vi "uA_Measurement_kit_v2_none_log.vi"() -> ()   [LabVIEW 2017]
uses:
  Range_Shunt_selector.ctl
  <vilib>/Utility/file.llb/Write Delimited Spreadsheet (string).vi
  <vilib>/Waveform/WDTFileIO.llb/ Write Waveform to File.vi
  <vilib>/Waveform/WDTFileIO.llb/Read Waveform from File.vi
  <vilib>/Utility/config.llb/Write Key (I32).vi
  <vilib>/Utility/config.llb/Write Key (Boolean).vi
  <vilib>/Utility/config.llb/Read Key (I32).vi
  <vilib>/Utility/config.llb/Read Key (Boolean).vi
  <vilib>/measure/madcrms.llb/Basic Averaged DC-RMS for 1 Chan.vi
  <resource>/objmgr/daqmx.rc
  <vilib>/Utility/config.llb/NI_LVConfig.lvlib
  <vilib>/measure/NI_MAPro.lvlib
panel:
  out "first_time":timestamp
  out "Ver":string
  out "Samples":i32=20000
  out "error out 3":errorcluster
  out "PhysicalChanName":tag
  out "DEV SN":u32 format="%.0x"
  out "mARange":dbl
  out "Boolean":bool
  out "DevSerialNum":u32
  in  "uA_bank0":dbl=1.5 format="%#_13g"
  out "Task out":refnum<k21>="Stop"
  out "Sample rate":dbl=20000.0 format="%#_13g"
  out "Clear":bool=TRUE
  out "seconds since 1Jan1904":timestamp
  in  "Tab Control":enum32{"Current Tracking", "Logging"}(tab)
  out "Total Time":i32
  in  "Sampling Rate":T1(ring)
  out "out_range":bool
  in  "Save setting":bool
  out "PW_Source":bool
  out "EX_IN_INdicator":bool
  out "Lable.Unit_VOl_MA_UA":string
  in  "Ext PW Vol Monitor":bool
  out "POWER ON_OFF":bool
  out "vbat_lb":dbl format="%#_4f"
  in  "bypass Shunt":bool
  in  "Internal PW":bool
  in  "USB":tag="Dev1"
  out "schematic":bool
  in  "Save":bool
  in  "Load":bool
  in  "Calib":bool
  in  "Power ON/OFF":bool
  in  "Profile":enum16{"SAM", "DIANA", "Hi-POWER", "Other..."}(ring)
  in  "Take Picture":bool
  in  "Orginal":bool
  in  "Clear Graph":bool
  in  "ZOOM M1M2":bool
  in  "ZOOM -":bool
  in  "ZOOM +":bool
  in  "stop":bool
  out "Vbat":dbl format="%#.3f"
  in  "Measure":bool
  in  "Range - Shunts":T2
  out "PW_Internal_Source":dbl
  out "Min":dbl
  out "Max":dbl
  out "Delta(s)":sgl
  in  "Center":bool
  out "Avg":dbl
  out "Waveform_main":waveform(sgl)(graph)
  out "Waveform_sub":waveform(dbl)(graph)
  out "Average (uA)":dbl caption="Average (mA)" format="%#_6f"
  in  "Vout  - Vbat profile":enum16{"3.8VDC", "2.9VDC", "By Pass", "4.0VDC"}(ring)=enum."2.9VDC" caption="Vout  - Vbat"
  # "Vbat"
  # "Vdut- Vbat"
  # "DUT"
  # "µPower kit for Wear OS Dev"
  # "Rs"
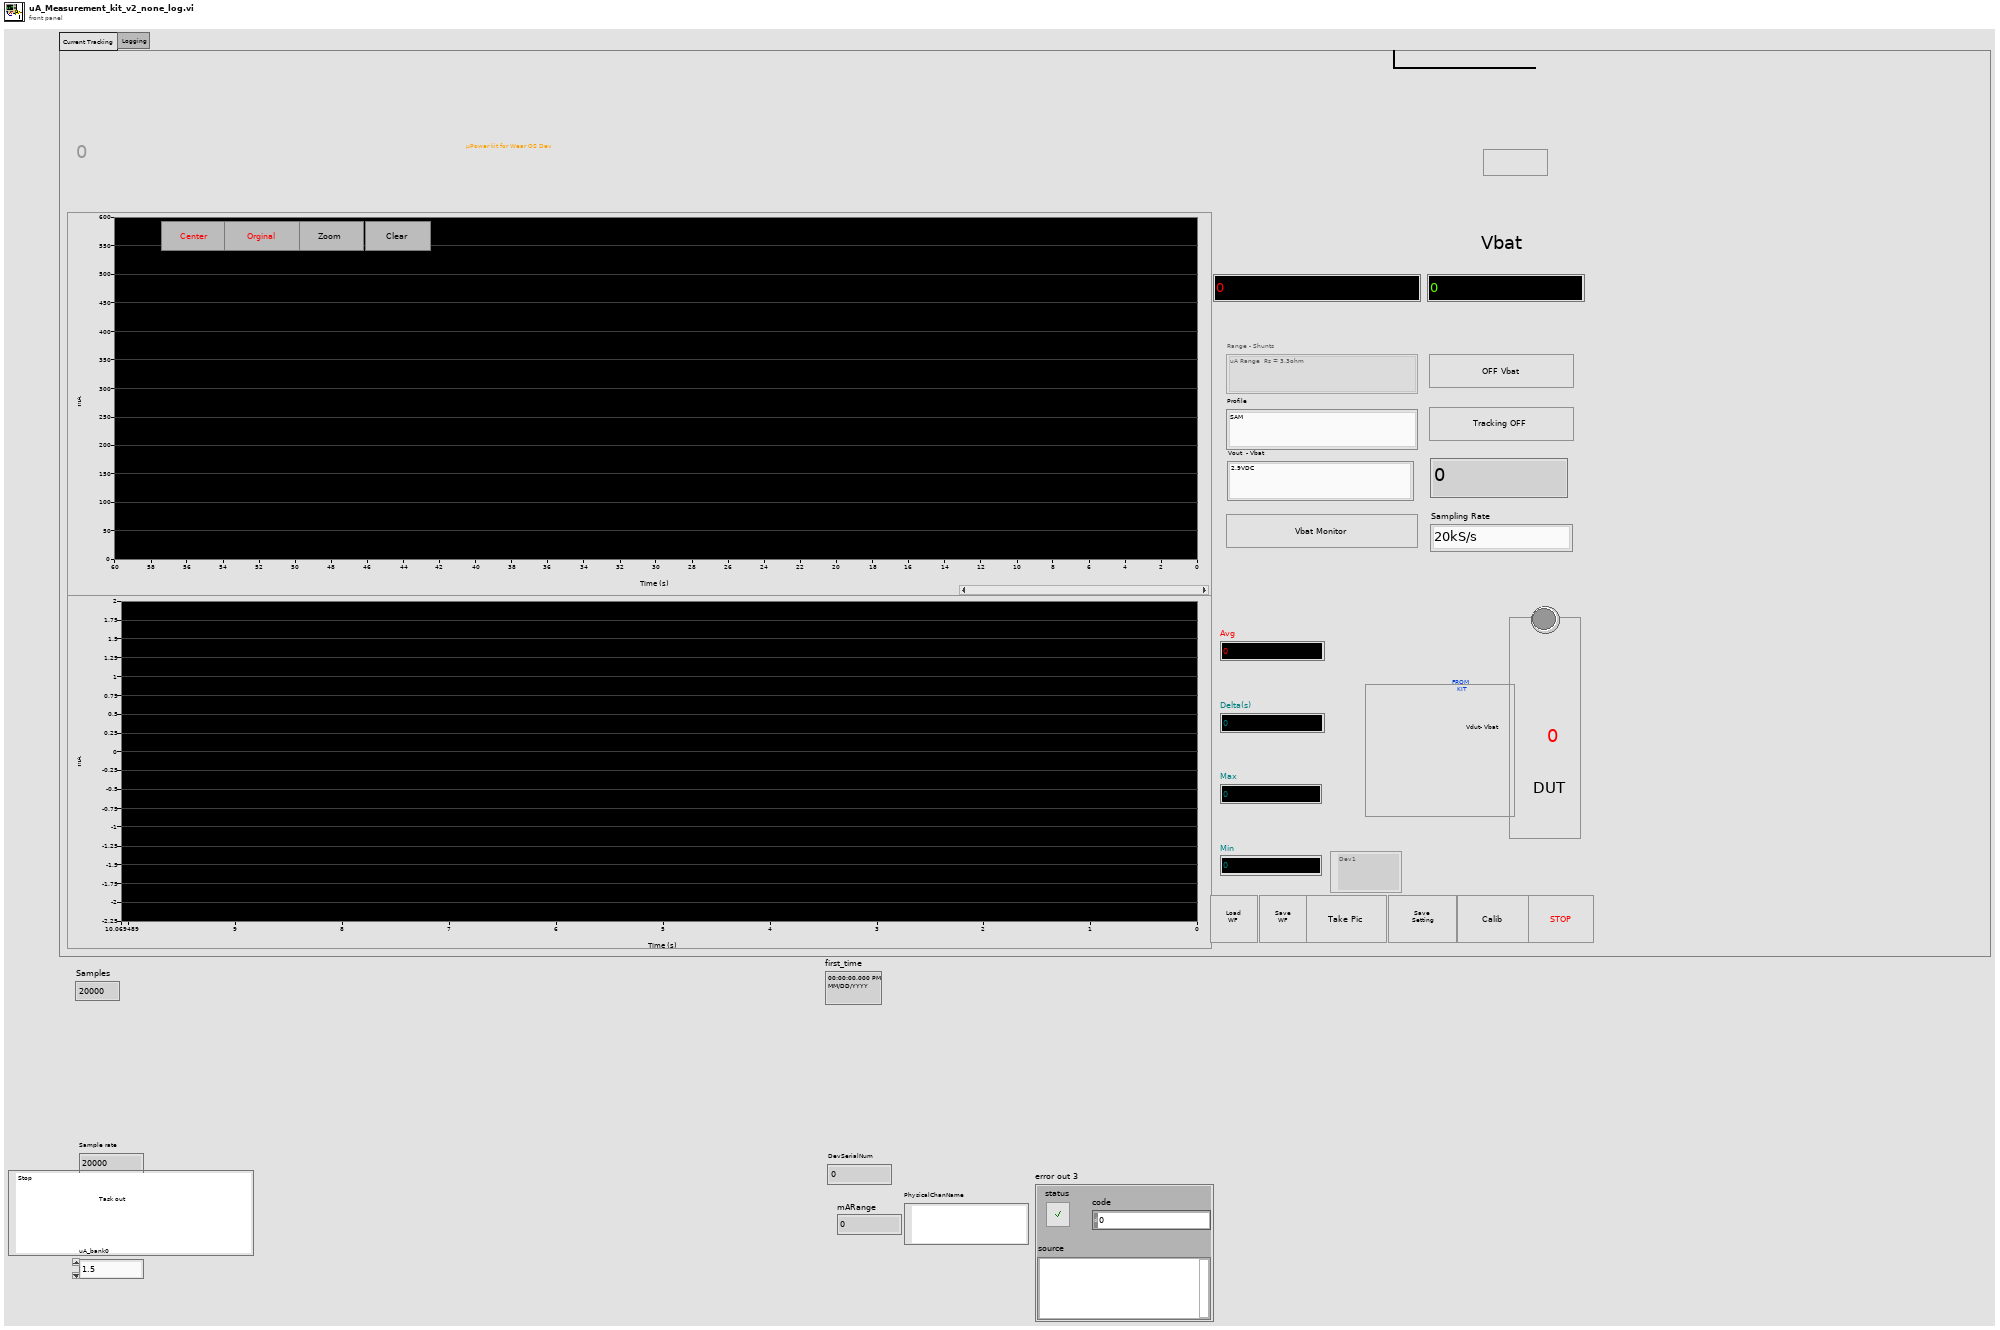
[diagram p1: front panel]
types:
  T1 = enum16{"20kS/s", "10kS/s", "5kS/s", "2kS/s", "1kS/s", "500S/s", "100S/s"}
  T2 = typedef "Range_Shunt_selector.ctl" = enum16{"uA Range  Rs = 3.3ohm", "mA Range Rs = 3.3ohm", "mA Range Rs = 1ohm", "mA Range Rs = 1ohm - X2"}
  T3 = enum8{"Enabled", "Disabled", "Disabled and Grayed Out"}
  T4 = enum16{"open", "replace", "create", "open or create", "replace or create", "replace or create with confirmation"}
  T5 = typedef "NI_LVConfig.lvlib/Config Data RefNum.ctl" = refnum<k1>
  T6 = enum16{"Internal PW Source", "External PW Source"}
  T7 = enum16{"Turn On bypass - Off Shunt", "Turn Off bypass - On Shunt"}
  T8 = typedef "LVCursorListTypeDef.ctl" = cluster{"Name":string, "Color":u32, "Style":u8, "Point Style":u8, "Name Visible":bool, "Allow Drag":bool, "Cursor Mode":u32, "Plot":i32, "Index":i32, "Position":cluster{"X":dbl, "Y":dbl}, "X Scale":u32, "Y Scale":u32, "Watch Plots":i32[], "Watch All Plots":bool, "Plot Area":i32, "Label Offset":cluster{"X":dbl, "Y":dbl}}[]
  T9 = typedef "imagedata.ctl" = cluster{"image type":i32, "image depth":i32, "image":u8[], "mask":u8[], "colors":u32[], "Rectangle":cluster{"left":i16, "top":i16, "right":i16, "bottom":i16}}
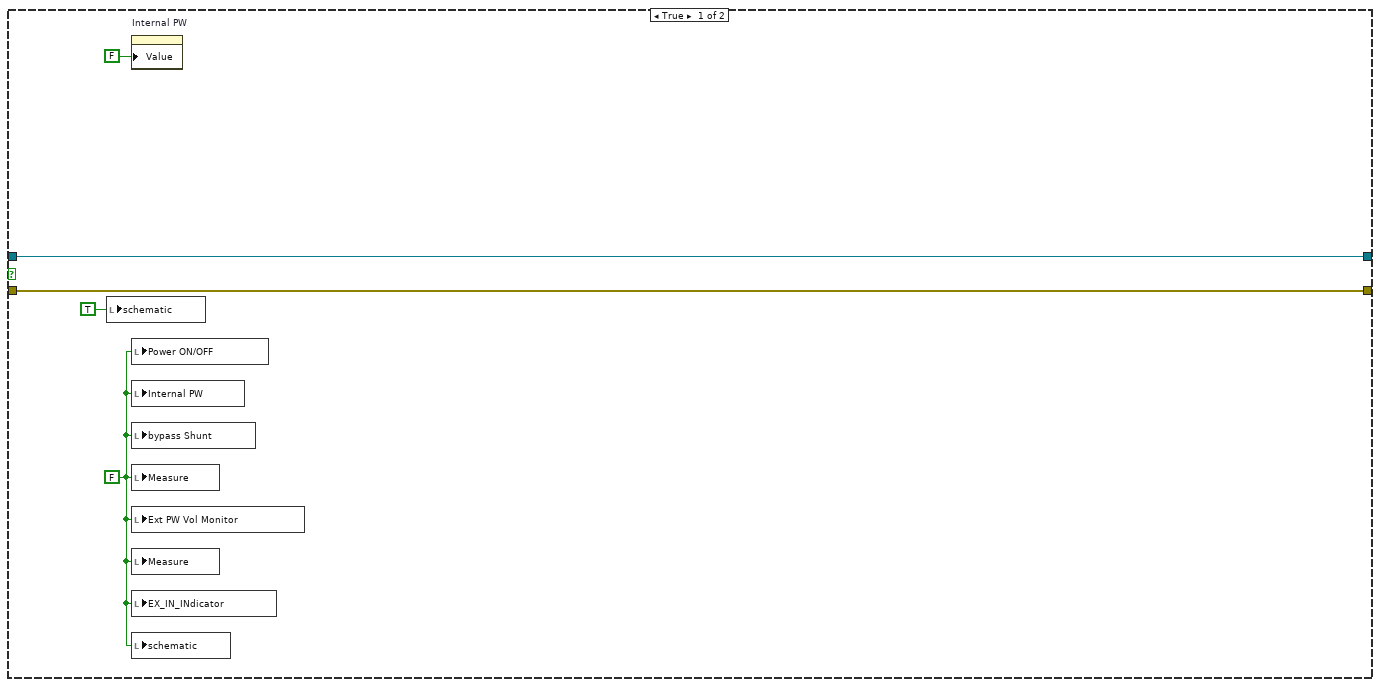
[diagram p3: hidden frame]
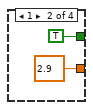
[diagram p4: hidden frame]
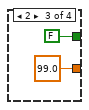
[diagram p5: hidden frame]
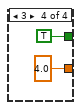
[diagram p6: hidden frame]
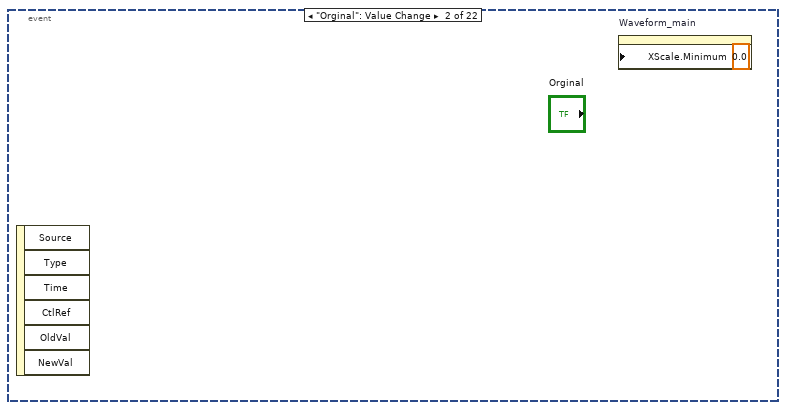
[diagram p12: hidden frame]
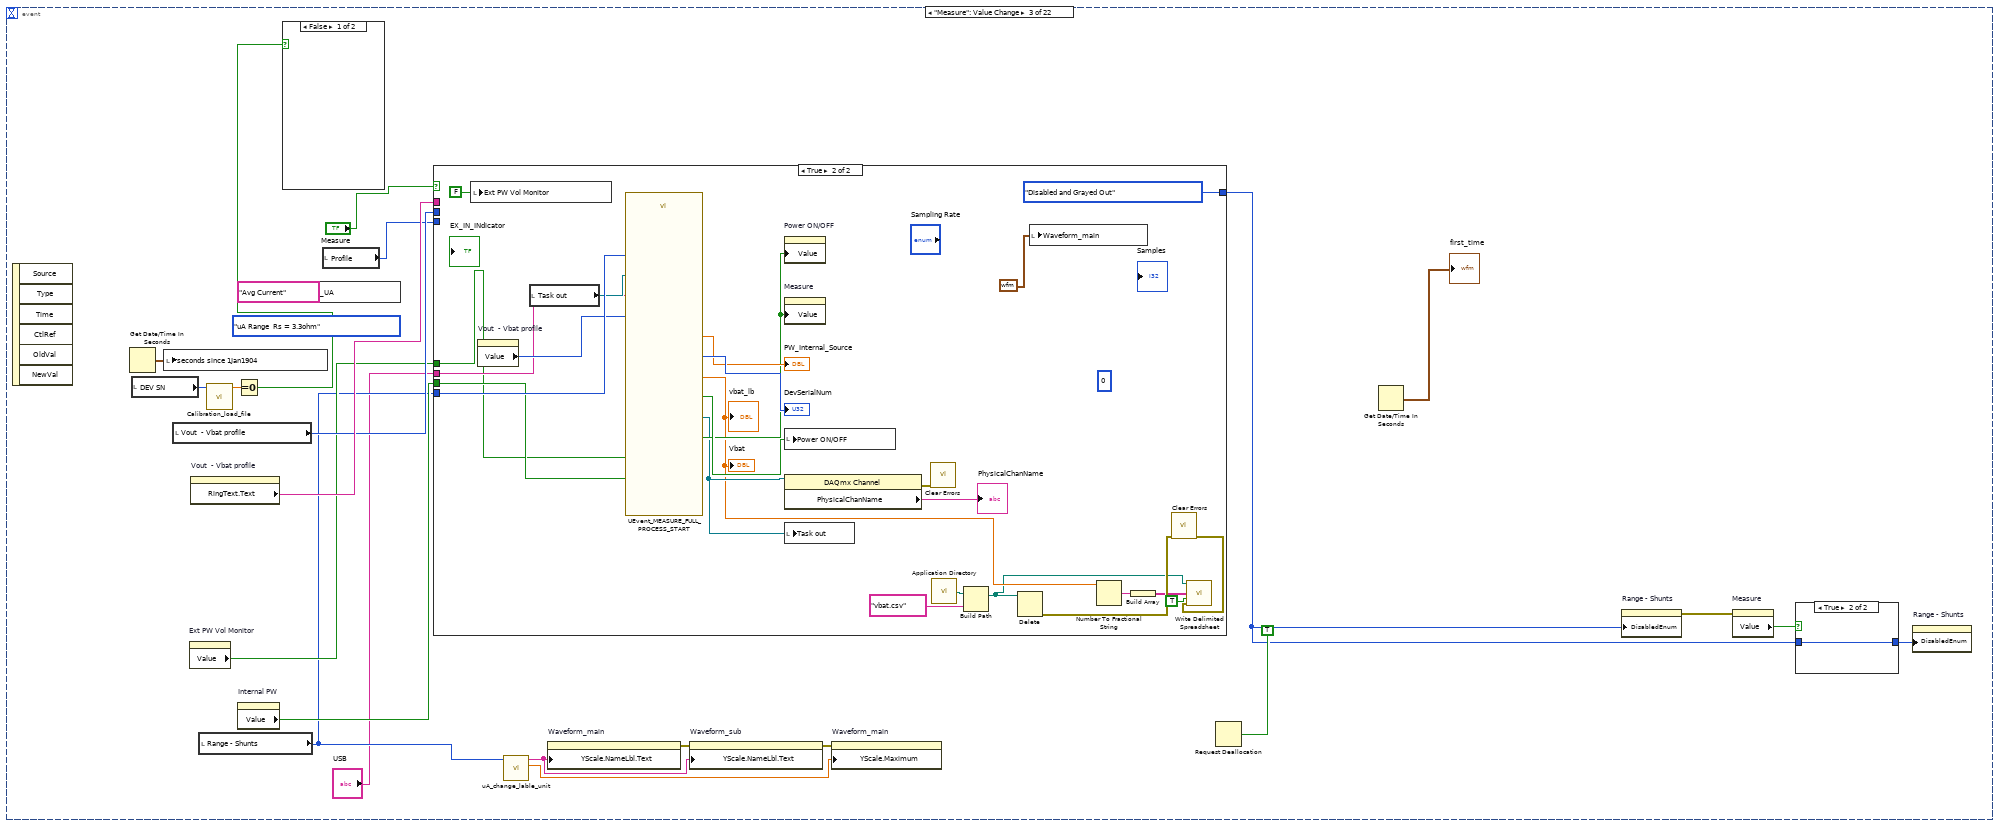
[diagram p13: hidden frame]
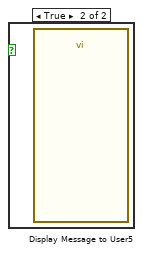
[diagram p14: hidden frame]
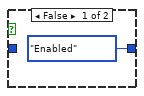
[diagram p15: hidden frame]
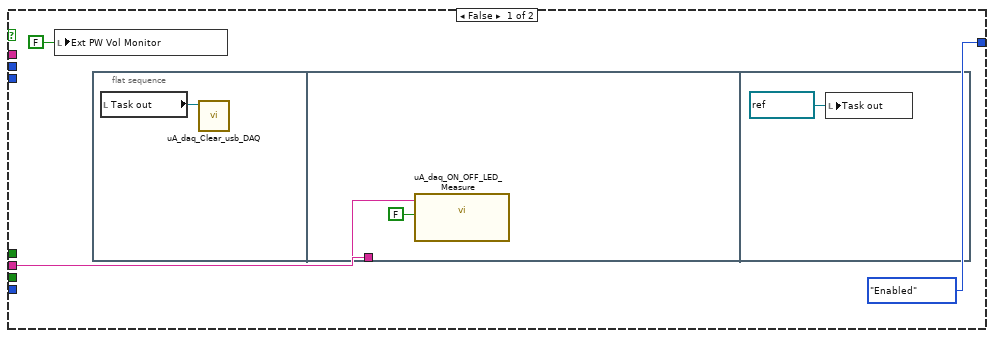
[diagram p16: hidden frame]
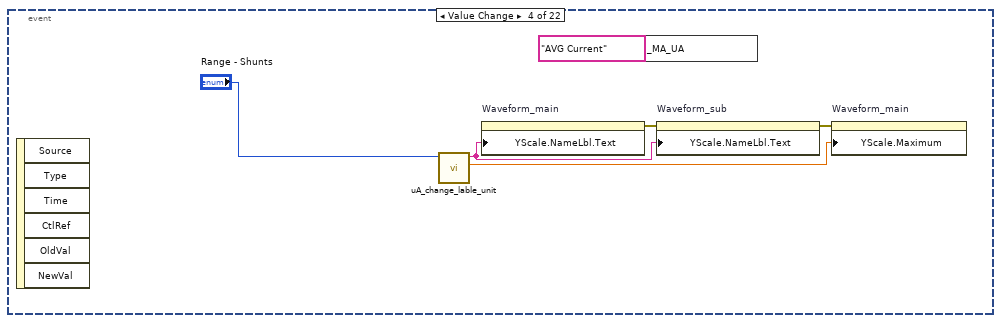
[diagram p17: hidden frame]
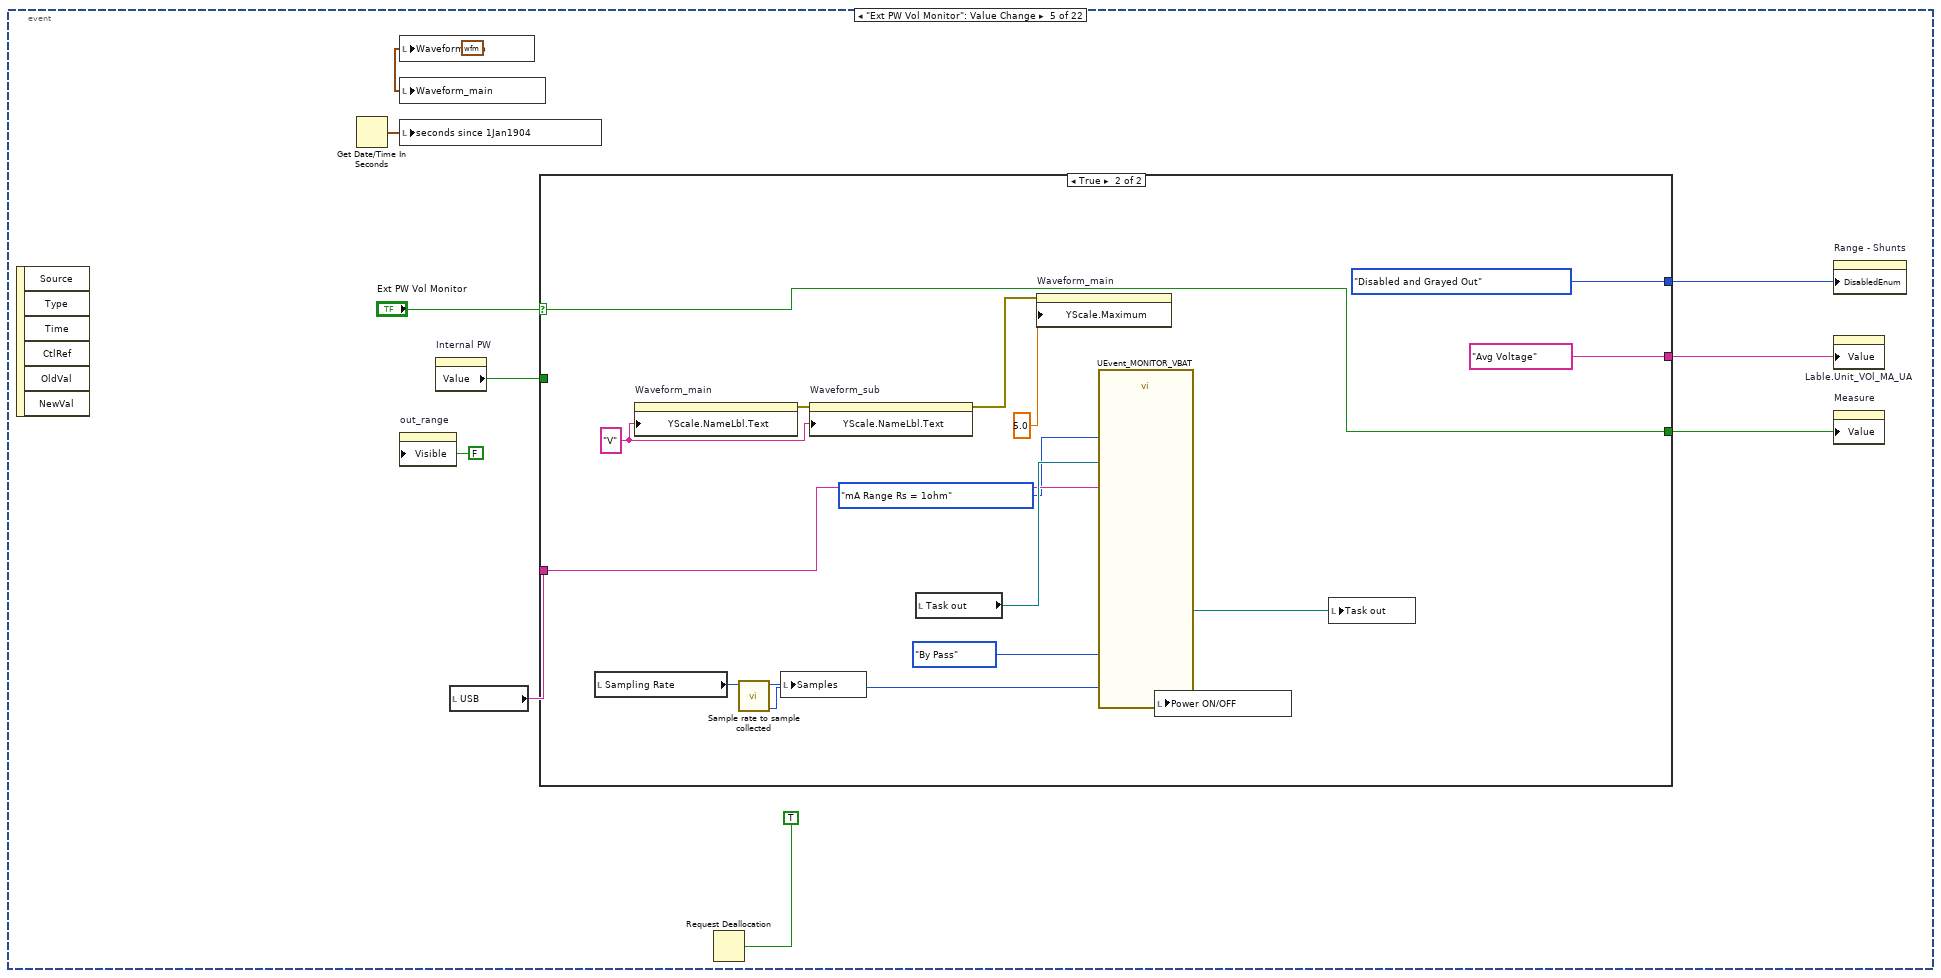
[diagram p18: hidden frame]
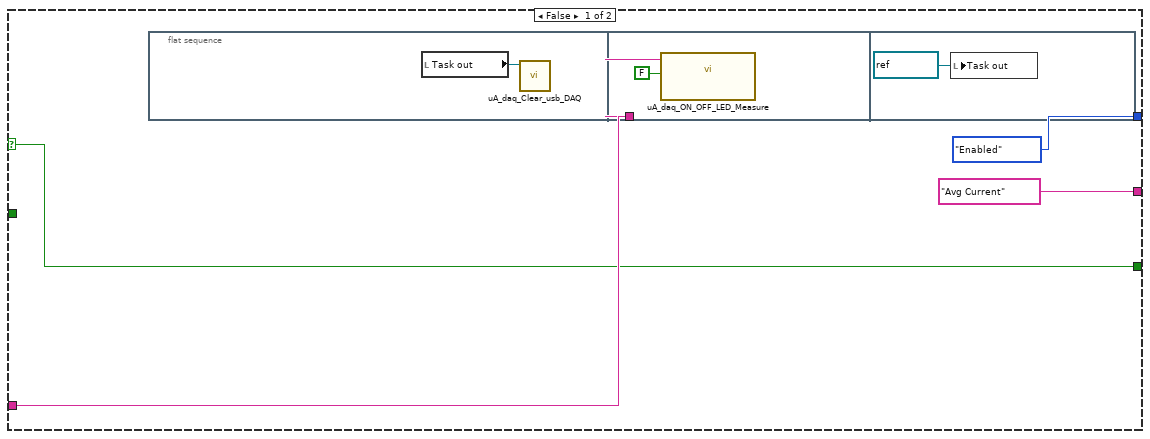
[diagram p19: hidden frame]
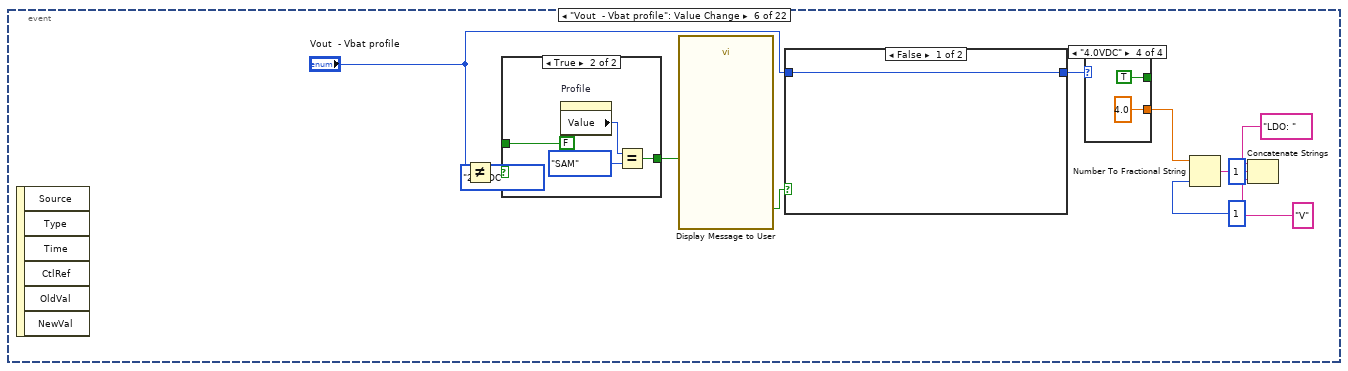
[diagram p20: hidden frame]
diagram:
  w2 = 24164516  # 1200s
  n1 = flat-sequence {
    tunnel: [w45] -> w5
    tunnel: [w48] -> w4
    frame #0 {
      w15 = TRUE ("s")
      w26 = FALSE ("Power ON/OFF")
      w45 = refnum<k21> "Stop" ("task out")
      n2 = property class="DAQmx System"() -> (error out=w39:errorcluster, "Device Names"=w40:tag[])  [unwired: 2 in, 1 out]
      n3 = property on="Range - Shunts" class="Enum (strict)"("DisabledEnum"=T3."Enabled" ("Disabled")) -> (error out=w8:errorcluster)  [unwired: 2 in, 1 out]
      n4 = local write "Vout  - Vbat profile"(enum16{"3.8VDC", "2.9VDC", "By Pass", "4.0VDC"}."By Pass" ("Vout  - Vbat profile")) -> ()
      n5 = local write "Profile"(enum16{"SAM", "DIANA", "Hi-POWER", "Other..."}."Hi-POWER" ("Profile")) -> ()
      n6 = for {
        tunnel: w40 -> [w102] mode=indexing
        shift-right: [w106] -> _
        shift-left: w39 -> [w107]
        tunnel: [w102] -> w38
        tunnel: [w101] -> w20
        stop <- w103 stop-if-true
        n7 = property class="DAQmx Device"(error in=w107, "Active Device"=w102) -> (error out=w106:errorcluster, "DevSerialNum"=w101:u32, "DevIsSimulated"=w105:bool)  [unwired: 1 in, 1 out]
        n8 = Equal?(x=w105, y=FALSE) -> (x = y?=w103:bool)
      }
      "DEV SN" <- w20
      n9 = local write "Power ON/OFF"(w26) -> ()
      n10 = local write "POWER ON_OFF"(w26) -> ()
      n11 = Select(t="Average (mA)" ("Caption.Text"), s=w15, f="Average (uA)" ("Caption.Text")) -> (s? t:f=w18:string)
      n12 = call <vilib>:"Application Directory.vi"() -> ("Application Directory"=w33:path)
      n13 = Select(t="mA" ("Caption.Text"), s=w15, f="uA" ("Caption.Text")) -> (s? t:f=w17:string)
      n14 = property on="out_range" class="Bool (strict)"(error in=w8, "Visible"=FALSE) -> (error out=w11:errorcluster)  [unwired: 1 in, 1 out]
      n15 = Build Path(base path=w33, name or relative path="Setting.cfg") -> (appended path=w31:path)
      n16 = property on="Average (uA)" class="DigNum (strict)"("Caption.Text"=w18) -> ()  [unwired: 2 in, 2 out]
      n17 = property on="Waveform_sub" class="WFGraph (strict)"("YScale.NameLbl.Text"=w17) -> ()  [unwired: 2 in, 2 out]
      n18 = property on="Waveform_main" class="WFGraph (strict)"("YScale.NameLbl.Text"=w17) -> ()  [unwired: 2 in, 2 out]
      n19 = call <vilib>:"Open Config Data.vi"("configuration file path"=w31) -> ("error out"=w27:errorcluster, "file created?"=w34:bool, "refnum"=w30:T5)  [unwired: 8 in]
      n20 = property on="Ext PW Vol Monitor" class="Bool (strict)"(error in=w11, "Value"=FALSE ("Record uA & Vbat")) -> (error out=w10:errorcluster)  [unwired: 1 in, 1 out]
      n21 = case shown="False" w34 {
        tunnel: w27 -> [w62 w92]
        tunnel: [w62 w87] -> w28
        tunnel: [w61 w86] -> w29
        tunnel: w30 -> [w61 w75]
        frame True {
          w60 = FALSE ("Measure")
          n22 = local write "schematic"(TRUE ("schematic")) -> ()
          n23 = property on="Internal PW" class="Bool (strict)"("Value"=FALSE ("Internal PW")) -> ()  [unwired: 2 in, 2 out]
          n24 = local write "Power ON/OFF"(w60) -> ()
          n25 = local write "Internal PW"(w60) -> ()
          n26 = local write "bypass Shunt"(w60) -> ()
          n27 = local write "Measure"(w60) -> ()
          n28 = local write "Ext PW Vol Monitor"(w60) -> ()
          n29 = local write "Measure"(w60) -> ()
          n30 = local write "EX_IN_INdicator"(w60) -> ()
          n31 = local write "schematic"(w60) -> ()
        }
        frame False {
          (unwired) FALSE ("Visible")
          w63 = TRUE
          w76 = "SETTING" ("section")
          n32 = Not(x=w63) -> ()  [unwired: 1 out]
          n33 = local write "Internal PW"(w63) -> ()
          n34 = local write "EX_IN_INdicator"(w63) -> ()
          n35 = local write "Vout  - Vbat profile"(enum16{"3.8VDC", "2.9VDC", "By Pass", "4.0VDC"}."By Pass" ("Vout  - Vbat profile")) -> ()
          n36 = local write "Profile"(enum16{"SAM", "DIANA", "Hi-POWER", "Other..."}."Hi-POWER" ("Profile")) -> ()
          n37 = call-poly <vilib>:"Read Key.vi"("section"=w76, "error in (no error)"=w92, "key"="Range - Shunts", "refnum"=w75) -> ("error out"=w91:errorcluster, "refnum out"=w78:T5)  [unwired: 4 in, 2 out]
          n38 = local write "Range - Shunts"(Range_Shunt_selector."mA Range Rs = 1ohm" ("Range - Shunts")) -> ()
          n39 = call-poly <vilib>:"Read Key.vi"("section"=w76, "error in (no error)"=w91, "key"="Profile", "refnum"=w78) -> ("error out"=w90:errorcluster, "refnum out"=w77:T5)  [unwired: 4 in, 2 out]
          n40 = call-poly <vilib>:"Read Key.vi"("section"=w76, "error in (no error)"=w90, "key"="Vout  - Vbat profile", "refnum"=w77) -> ("error out"=w89:errorcluster, "value"=w67:i32, "refnum out"=w79:T5)  [unwired: 4 in, 1 out]
          n41 = case shown="0, Default" w67 {
            tunnel: [3.8 2.9 99.0 4.0] -> w71
            tunnel: [TRUE ("Visible") TRUE ("Visible") FALSE ("Visible") TRUE ("Visible")] -> _
            frame 0, Default {
            }
            frame 1 {
            }
            frame 2 {
            }
            frame 3 {
            }
          }
          n42 = call-poly <vilib>:"Read Key.vi"("section"=w76, "error in (no error)"=w89, "key"="Internal PW", "refnum"=w79) -> ("error out"=w88:errorcluster, "refnum out"=w80:T5)  [unwired: 4 in, 2 out]
          n43 = call-poly <vilib>:"Read Key.vi"("section"=w76, "error in (no error)"=w88, "key"="bypass Shunt", "refnum"=w80) -> ("error out"=w87:errorcluster, "value"=w74:bool, "refnum out"=w86:T5)  [unwired: 4 in, 1 out]
          n44 = local write "bypass Shunt"(w74) -> ()
          n45 = Number To Fractional String(number=w71, width (-)=i16 1, precision (6)=i16 1) -> (F-format string=w68:string)  [unwired: 1 in]
          n46 = Concatenate Strings("LDO: " ("string"), w68, "V" ("string")) -> ()  [unwired: 1 out]
        }
      }
      n47 = local write "USB"(w38) -> ()
      n48 = property on="out_range" class="Bool (strict)"(error in=w10, "Visible"=FALSE) -> (error out=w9:errorcluster)  [unwired: 1 in, 1 out]
      n49 = call "Calibration_load_file.vi"("DEV SN"=w20) -> ("Calib value-mA"=→"mARange":dbl, "Calib value-uA"=w21:dbl)  [unwired: 8 in]
      n50 = local write "uA_bank0"(w21) -> ()
      n51 = call <vilib>:"Application Directory.vi"() -> ("Application Directory"=w47:path)
      n52 = call "uA_build_version.vi"("error in (no error)"=w9, "name or relative path"="uPower_kit_wear_os.exe", "path"=w47) -> ("error out"=w44:errorcluster, "FileVersion"=w43:string)  [unwired: 6 in, 1 out]
      n53 = case shown="Error" w44 {
        selector: w44 -> [_ w110]
        tunnel: w43 -> [w108 _]
        tunnel: [w108 "" ("FileVersion")] -> w42
        frame No Error {
        }
        frame Error {
          n54 = call <vilib>:"Clear Errors.vi"("error in (no error)"=w110) -> ()  [unwired: 5 in, 2 out]
        }
      }
      "Ver" <- w42
      n55 = local write "Measure"(FALSE ("Measure")) -> ()
      n56 = local write "schematic"(TRUE ("schematic")) -> ()
      n57 = disable-structure shown="Disabled" {
        frame Disabled {
          n58 = call <vilib>:"Application Directory.vi"() -> ("Application Directory"=w57:path)
          n59 = Build Path(base path=w57, name or relative path="datalog.dlog" ("pattern label")) -> (appended path=w55:path)
          n60 = Open/Create/Replace File(file path (use dialog)=w55, operation (0:open)=T4."replace or create", access (0:read/write)=enum16{"read/write", "read-only", "write-only"}."write-only") -> ()  [unwired: 3 in, 3 out]
        }
        frame Enabled {
        }
      }
      n61 = call <vilib>:"Close Config Data.vi"("error in (no error)"=w28, "refnum"=w29) -> ()  [unwired: 8 in, 2 out]
      n62 = Obtain Queue(name (unnamed)="Data", element data type=waveform(sgl) {"t0"=timestamp(0 s since 1904-01-01), "dt"=1.0, "Y"=[]} ("Waveform Chart 2")) -> (queue out=w48:refnum<queue>)  [unwired: 3 in, 2 out]
      "Clear" <- FALSE ("Clear")
      "Sample rate" <- 20000.0 ("Sample rate")
      "Task out" <- w45
    }
  }
  n63 = Multiply(x=w2, y=4) -> (x*y=w1:i32)
  n64 = while {
    stop <- FALSE stop-if-true
    n65 = event shown="[0] Timeout" {
      selector: _ -> [_ _ _ _ _ _ _ _ _ _ _ _ _ _ _ _ _ _ _ _ _ _]
      dyn-events: _ -> [_ _ _ _ _ _ _ _ _ _ _ _ _ _ _ _ _ _ _ _ _ _]
      timeout: 400 -> [_ _ _ _ _ _ _ _ _ _ _ _ _ _ _ _ _ _ _ _ _ _]
      event Timeout {
        n66 = event-data() -> ()  [unwired: 1 in, 3 out]
        n67 = disable-structure shown="Disabled" {
          frame Disabled {
            n68 = local read "Task out"() -> (w114:refnum<k21>)
            n69 = Equal?(x=w114, y=refnum<k21> "Stop") -> (x = y?=w115:bool)
            n70 = case shown="False" w115 {
              frame True {
              }
              frame False {
                n71 = local read "seconds since 1Jan1904"() -> (w120:timestamp)
                n72 = local read "first_time"() -> (w118:timestamp)
                n73 = Get Date/Time In Seconds() -> (seconds since 1Jan1904=w119:timestamp)
                n74 = Subtract(x=w119, y=w118) -> (x-y=→"Total Time":dbl)
                n75 = Subtract(x=w119, y=w120) -> (x-y=w123:dbl)
                n76 = Greater Or Equal?(x=w123, y=60.0) -> (x >= y?=w121:bool)
                n77 = case shown="True" w121 {
                  tunnel: w119 -> [_ _]
                  frame False {
                  }
                  frame True {
                    w140 = 5 items=["verify"=2, "reserve"=4, "commit"=3, "unreserve"=5, "abort"=6] ("action")
                    n78 = Get Date/Time In Seconds() -> (seconds since 1Jan1904=→"seconds since 1Jan1904":timestamp)
                    n79 = local read "Task out"() -> (w154:refnum<k21>)
                    n80 = call <vilib>:"DAQmx Stop Task.vi"("task/channels in"=w154) -> ("task out"=w144:refnum<k21>, "error out"=w142:errorcluster)  [unwired: 13 in]
                    n81 = call <vilib>:"DAQmx Control Task.vi"("task/channels in"=w144, "action"=w140, "error in"=w142) -> ("task out"=w143:refnum<k21>, "error out"=w141:errorcluster)  [unwired: 11 in]
                    n82 = call <vilib>:"DAQmx Clear Task.vi"("task in"=w143, "error in"=w141) -> ("error out"=w136:errorcluster)  [unwired: 13 in]
                    n83 = case shown="No Error" w136 {
                      selector: w136 -> [w157 w159]
                      tunnel: [w157 w159] -> w135
                      frame No Error {
                        n84 = Wait (ms)(milliseconds to wait=u32 100) -> ()  [unwired: 1 out]
                        n85 = local write "Task out"(refnum<k21> "Stop" ("Task out")) -> ()
                      }
                      frame Error {
                      }
                    }
                    n86 = local read "USB"() -> (w146:tag)
                    n87 = call <vilib>:"Clear Errors.vi"("error in (no error)"=w135) -> ("error out"=w153:errorcluster)  [unwired: 5 in, 1 out]
                    n88 = property on="Range - Shunts" class="Enum (strict)"() -> ("Value"=w150:T2)  [unwired: 2 in, 2 out]
                    n89 = call "uA_daq_Read_Battery_Voltage.vi"("error in"=w153, "USB DAQ"=w146) -> ("error out"=w151:errorcluster, "Battery_Voltage"=w152:dbl)  [unwired: 8 in]
                    n90 = local write "PW_Internal_Source"(w152) -> ()
                    n91 = call "uA_daq_Read_DUT_Voltage.vi"("error in"=w151, "USB DAQ"=w146) -> ("error out"=w139:errorcluster, "DUT_Voltage"=w124:dbl)  [unwired: 8 in]
                    n92 = local write "Vbat"(w124) -> ()
                    n93 = call <vilib>:"Application Directory.vi"() -> ("Application Directory"=w129:path)
                    n94 = Number To Fractional String(number=w124) -> (F-format string=w126:string)  [unwired: 3 in]
                    n95 = Build Path(base path=w129, name or relative path="vbat.csv" ("pattern label")) -> (appended path=w128:path)
                    n96 = Build Array(w126) -> (w125:string[])
                    n97 = local read "Sampling Rate"() -> (w132:T1)
                    n98 = property on="Ext PW Vol Monitor" class="Bool (strict)"() -> ("Value"=w147:bool)  [unwired: 2 in, 2 out]
                    n99 = call-poly <vilib>:"Write Delimited Spreadsheet.vi"("file path (dialog if empty)"=w128, "1D data"=w125, "append to file? (new file:F)"=TRUE) -> ()  [unwired: 11 in, 2 out]
                    n100 = call "Sample rate to sample collected.vi"("Sampling Rate _menu"=w132) -> ("Sample_rate"=w131:u32, "Sample"=w133:i32)  [unwired: 9 in]
                    n101 = for {
                      N: 3 -> [_]
                      tunnel: w150 -> [w167]
                      tunnel: [w166] -> w149
                      tunnel: w146 -> [w165]
                      tunnel: enum16{"Streaming", "Read All", "Stop"}."Streaming" ("Acquire Mode") -> [w163]
                      tunnel: w139 -> [w164]
                      tunnel: [w162] -> w145
                      tunnel: w131 -> [w160]
                      stop <- w161 continue-if-true
                      n102 = call "uA_daq_Re_Init_daq_follow_input.vi"("rate"=w160, "error in (no error)"=w164, "Acquire Mode"=w163, "USB"=w165, "Range_shunt"=w167) -> ("error out"=w162:errorcluster, "Refnum out"=w166:refnum<k21>)  [unwired: 5 in]
                      n103 = Unbundle By Name(w162) -> ("status"=w161:bool)
                    }
                    n104 = local write "Samples"(w133) -> ()
                    n105 = call "uA_DAQ_Init_Monitor_Stream_vbat_selector.vi"("Sample rate"=w131, "error in (no error)"=w145, "USB"=w146, "Ext PW Vol Monitor"=w147, "Refnum in"=w149) -> ("error out"=w134:errorcluster, "Refnum out"=w148:refnum<k21>)  [unwired: 5 in]
                    n106 = call <vilib>:"Clear Errors.vi"("error in (no error)"=w134) -> ()  [unwired: 5 in, 2 out]
                    n107 = local write "Task out"(w148) -> ()
                  }
                }
              }
            }
          }
          frame Enabled {
          }
        }
        n108 = local read "Vbat"() -> (w113:dbl)
        n109 = local write "vbat_lb"(w113) -> ()
      }
      event "Orginal": Value Change {
        n110 = event-data() -> ()  [unwired: 1 in, 6 out]
        n111 = property on="Waveform_main" class="WFGraph (strict)"("XScale.Minimum"=0.0 ("X Scale.Range:Minimum")) -> ()  [unwired: 2 in, 2 out]
      }
      event "Measure": Value Change {
        (unwired) Range_Shunt_selector."uA Range  Rs = 3.3ohm" ("Range - Shunts")
        n112 = event-data() -> ()  [unwired: 1 in, 6 out]
        n113 = Get Date/Time In Seconds() -> (seconds since 1Jan1904=w190:timestamp)
        n114 = local read "DEV SN"() -> (w172:u32)
        n115 = local write "seconds since 1Jan1904"(w190) -> ()
        n116 = local read "Vout  - Vbat profile"() -> (w187:enum16{"3.8VDC", "2.9VDC", "By Pass", "4.0VDC"})
        n117 = property on="Ext PW Vol Monitor" class="Bool (strict)"() -> ("Value"=w180:bool)  [unwired: 2 in, 2 out]
        n118 = property on="Vout  - Vbat profile" class="Enum (strict)"() -> ("RingText.Text"=w188:string)  [unwired: 2 in, 2 out]
        n119 = local read "Range - Shunts"() -> (w178:T2)
        n120 = call "Calibration_load_file.vi"("DEV SN"=w172) -> ("Calib value-uA"=w171:dbl)  [unwired: 8 in, 1 out]
        n121 = Equal To 0?(x=w171) -> (x = 0?=w170:bool)
        n122 = property on="Internal PW" class="Bool (strict)"() -> ("Value"=w181:bool)  [unwired: 2 in, 2 out]
        n123 = local write "Lable.Unit_VOl_MA_UA"("Avg Current" ("Lable.Unit_VOl_MA_UA")) -> ()
        n124 = case shown="False" w170 {
          frame False {
          }
          frame True {
            n125 = call "Display Message to User5"() -> ()  [unwired: 10 in, 2 out]
          }
        }
        n126 = local read "Profile"() -> (w186:enum16{"SAM", "DIANA", "Hi-POWER", "Other..."})
        n127 = case shown="True" "Measure" {
          tunnel: w188 -> [_ _]
          tunnel: w187 -> [_ _]
          tunnel: w186 -> [_ _]
          tunnel: w178 -> [_ w222]
          tunnel: w181 -> [_ w219]
          tunnel: "USB" -> [w195 w217]
          tunnel: w180 -> [_ w214]
          tunnel: [T3."Enabled" ("Disabled") T3."Disabled and Grayed Out" ("Disabled")] -> w174
          frame False {
            n128 = local write "Ext PW Vol Monitor"(FALSE ("Ext PW Vol Monitor")) -> ()
            n129 = flat-sequence {
              tunnel: w195 -> [w199]
              frame #0 {
                n130 = local read "Task out"() -> (w197:refnum<k21>)
                n131 = call "uA_daq_Clear_usb_DAQ.vi"("Refnum in"=w197) -> ()  [unwired: 11 in]
              }
              frame #1 {
                n132 = call "uA_daq_ON_OFF_LED_Measure.vi"("LED_meas"=FALSE ("Boolean"), "USB"=w199) -> ()  [unwired: 9 in, 1 out]
              }
              frame #2 {
                n133 = local write "Task out"(refnum<k21> "Stop" ("Refnum out")) -> ()
              }
            }
          }
          frame True {
            (unwired) u16 0 ("File_Record")
            n134 = local write "Ext PW Vol Monitor"(FALSE ("Ext PW Vol Monitor")) -> ()
            n135 = property on="Vout  - Vbat profile" class="Enum (strict)"() -> ("Value"=w220:enum16{"3.8VDC", "2.9VDC", "By Pass", "4.0VDC"})  [unwired: 2 in, 2 out]
            n136 = local read "Task out"() -> (w221:refnum<k21>)
            n137 = call "UEvent_MEASURE_FULL_PROCESS_START.vi"("Refnum in"=w221, "Range - Shunts"=w222, "Ext PW Vol Monitor"=w214, "USB"=w217, "Internal/external Power"=w219, "Vout  - Vbat profile"=w220) -> ("DevSerialNum"=→"DevSerialNum":u32, "Power ON/OFF"=w224:bool, "Refnum out"=w216:refnum<k21>, "Battery_Voltage"=→"PW_Internal_Source":dbl, "DUT_Voltage"=w203:dbl, "Measure indicator"=w218:bool)  [unwired: 3 in, 1 out]
            "Vbat" <- w203
            "vbat_lb" <- w203
            n138 = property on="Power ON/OFF" class="Bool (strict)"("Value"=w218) -> ()  [unwired: 2 in, 2 out]
            n139 = property on="Measure" class="Bool (strict)"("Value"=w218) -> ()  [unwired: 2 in, 2 out]
            n140 = local write "Power ON/OFF"(w224) -> ()
            n141 = property class="DAQmx Channel"(reference=w216) -> (error out=w213:errorcluster, "PhysicalChanName"=→"PhysicalChanName":tag)  [unwired: 1 in, 1 out]
            n142 = local write "Task out"(w216) -> ()
            n143 = call <vilib>:"Clear Errors.vi"("error in (no error)"=w213) -> ()  [unwired: 5 in, 2 out]
            n144 = call <vilib>:"Application Directory.vi"() -> ("Application Directory"=w209:path)
            n145 = Build Path(base path=w209, name or relative path="vbat.csv" ("pattern label")) -> (appended path=w202:path)
            n146 = Delete(path (use dialog)=w202) -> (error out=w210:errorcluster)  [unwired: 4 in, 2 out]
            n147 = local write "Waveform_main"(waveform(dbl) {"t0"=timestamp(0 s since 1904-01-01), "dt"=1.0, "Y"=[]} ("Waveform")) -> ()
            n148 = Number To Fractional String(number=w203) -> (F-format string=w206:string)  [unwired: 3 in]
            n149 = Build Array(w206) -> (w205:string[])
            n150 = call <vilib>:"Clear Errors.vi"("error in (no error)"=w210) -> ("error out"=w201:errorcluster)  [unwired: 5 in, 1 out]
            n151 = call-poly <vilib>:"Write Delimited Spreadsheet.vi"("file path (dialog if empty)"=w202, "1D data"=w205, "append to file? (new file:F)"=TRUE, "error in (no error)"=w201) -> ()  [unwired: 10 in, 2 out]
          }
        }
        n152 = call "uA_change_lable_unit.vi"("Range - Shunts"=w178) -> ("Y_scale"=w183:dbl, "unit"=w182:string)  [unwired: 8 in, 1 out]
        n153 = property on="Waveform_main" class="WFGraph (strict)"("YScale.NameLbl.Text"=w182) -> (error out=w185:errorcluster)  [unwired: 2 in, 1 out]
        n154 = property on="Waveform_sub" class="WFGraph (strict)"(error in=w185, "YScale.NameLbl.Text"=w182) -> (error out=w184:errorcluster)  [unwired: 1 in, 1 out]
        n155 = property on="Waveform_main" class="WFGraph (strict)"(error in=w184, "YScale.Maximum"=w183) -> ()  [unwired: 1 in, 2 out]
        n156 = Request Deallocation(TRUE ("flag")) -> ()
        n157 = Get Date/Time In Seconds() -> (seconds since 1Jan1904=→"first_time":timestamp)
        n158 = property on="Range - Shunts" class="Enum (strict)"("DisabledEnum"=w174) -> (error out=w177:errorcluster)  [unwired: 2 in, 1 out]
        n159 = property on="Measure" class="Bool (strict)"(error in=w177) -> ("Value"=w176:bool)  [unwired: 1 in, 2 out]
        n160 = case shown="True" w176 {
          tunnel: [T3."Enabled" ("Disabled") w193] -> w175
          tunnel: w174 -> [_ w193]
          frame False {
          }
          frame True {
          }
        }
        n161 = property on="Range - Shunts" class="Enum (strict)"("DisabledEnum"=w175) -> ()  [unwired: 2 in, 2 out]
      }
      event Value Change {
        n162 = event-data() -> ()  [unwired: 1 in, 6 out]
        n163 = call "uA_change_lable_unit.vi"("Range - Shunts"="Range - Shunts") -> ("Y_scale"=w229:dbl, "unit"=w228:string)  [unwired: 8 in, 1 out]
        n164 = property on="Waveform_main" class="WFGraph (strict)"("YScale.NameLbl.Text"=w228) -> (error out=w231:errorcluster)  [unwired: 2 in, 1 out]
        n165 = local write "Lable.Unit_VOl_MA_UA"("AVG Current" ("Lable.Unit_VOl_MA_UA")) -> ()
        n166 = property on="Waveform_sub" class="WFGraph (strict)"(error in=w231, "YScale.NameLbl.Text"=w228) -> (error out=w230:errorcluster)  [unwired: 1 in, 1 out]
        n167 = property on="Waveform_main" class="WFGraph (strict)"(error in=w230, "YScale.Maximum"=w229) -> ()  [unwired: 1 in, 2 out]
      }
      event "Ext PW Vol Monitor": Value Change {
        w234 = waveform(sgl) {"t0"=timestamp(0 s since 1904-01-01), "dt"=1.0, "Y"=[]} ("Waveform_main")
        n168 = event-data() -> ()  [unwired: 1 in, 6 out]
        n169 = Get Date/Time In Seconds() -> (seconds since 1Jan1904=w240:timestamp)
        n170 = local write "Waveform_sub"(w234) -> ()
        n171 = local write "Waveform_main"(w234) -> ()
        n172 = local write "seconds since 1Jan1904"(w240) -> ()
        n173 = property on="out_range" class="Bool (strict)"("Visible"=FALSE) -> ()  [unwired: 2 in, 2 out]
        n174 = property on="Internal PW" class="Bool (strict)"() -> ("Value"=w239:bool)  [unwired: 2 in, 2 out]
        n175 = local read "USB"() -> (w237:tag)
        n176 = case shown="True" "Ext PW Vol Monitor" {
          selector: "Ext PW Vol Monitor" -> [w244 w262]
          tunnel: w239 -> [_ _]
          tunnel: w237 -> [w245 w263]
          tunnel: [w244 w262] -> w236
          tunnel: ["Avg Current" ("Lable.Unit_VOl_MA_UA") "Avg Voltage" ("Lable.Unit_VOl_MA_UA")] -> w235
          tunnel: [T3."Enabled" ("Disabled") T3."Disabled and Grayed Out" ("Disabled")] -> w233
          frame False {
            n177 = flat-sequence {
              tunnel: w245 -> [w248]
              frame #0 {
                n178 = local read "Task out"() -> (w246:refnum<k21>)
                n179 = call "uA_daq_Clear_usb_DAQ.vi"("Refnum in"=w246) -> ()  [unwired: 11 in]
              }
              frame #1 {
                n180 = call "uA_daq_ON_OFF_LED_Measure.vi"("LED_meas"=FALSE ("Boolean"), "USB"=w248) -> ()  [unwired: 9 in, 1 out]
              }
              frame #2 {
                n181 = local write "Task out"(refnum<k21> "Stop" ("Refnum out")) -> ()
              }
            }
          }
          frame True {
            w261 = "V" ("Y Scale.Name Label.Text")
            n182 = local read "Sampling Rate"() -> (w253:T1)
            n183 = property on="Waveform_main" class="WFGraph (strict)"("YScale.NameLbl.Text"=w261) -> (error out=w258:errorcluster)  [unwired: 2 in, 1 out]
            n184 = call "Sample rate to sample collected.vi"("Sampling Rate _menu"=w253) -> ("Sample_rate"=w252:u32, "Sample"=w254:i32)  [unwired: 9 in]
            n185 = local write "Samples"(w254) -> ()
            n186 = property on="Waveform_sub" class="WFGraph (strict)"(error in=w258, "YScale.NameLbl.Text"=w261) -> (error out=w259:errorcluster)  [unwired: 1 in, 1 out]
            n187 = local read "Task out"() -> (w264:refnum<k21>)
            n188 = property on="Waveform_main" class="WFGraph (strict)"(error in=w259, "YScale.Maximum"=5.0 ("Y Scale.Range:Maximum")) -> ()  [unwired: 1 in, 2 out]
            n189 = call "UEvent_MONITOR_VBAT.vi"("Vout  - Vbat profile"=enum16{"3.8VDC", "2.9VDC", "By Pass", "4.0VDC"}."By Pass", "Sample rate"=w252, "USB"=w263, "Range - Shunts"=Range_Shunt_selector."mA Range Rs = 1ohm", "Refnum in"=w264) -> ("Refnum out"=w256:refnum<k21>, "Power ON/OFF"=w265:bool)  [unwired: 1 in, 4 out]
            n190 = local write "Power ON/OFF"(w265) -> ()
            n191 = local write "Task out"(w256) -> ()
          }
        }
        n192 = Request Deallocation(TRUE ("flag")) -> ()
        n193 = property on="Range - Shunts" class="Enum (strict)"("DisabledEnum"=w233) -> ()  [unwired: 2 in, 2 out]
        n194 = property on="Lable.Unit_VOl_MA_UA" class="Str"("Value"=w235) -> ()  [unwired: 2 in, 2 out]
        n195 = property on="Measure" class="Bool (strict)"("Value"=w236) -> ()  [unwired: 2 in, 2 out]
      }
      event "Vout  - Vbat profile": Value Change {
        n196 = event-data() -> ()  [unwired: 1 in, 6 out]
        n197 = Not Equal?(x="Vout  - Vbat profile", y=enum16{"3.8VDC", "2.9VDC", "By Pass", "4.0VDC"}."2.9VDC" ("Vout  - Vbat profile")) -> (x != y?=w278:bool)
        n198 = case shown="True" w278 {
          tunnel: [w289 w290] -> w276
          tunnel: FALSE -> [w289 _]
          frame False {
          }
          frame True {
            n199 = property on="Profile" class="Enum (strict)"() -> ("Value"=w292:enum16{"SAM", "DIANA", "Hi-POWER", "Other..."})  [unwired: 2 in, 2 out]
            n200 = Equal?(x=w292, y=enum16{"SAM", "DIANA", "Hi-POWER", "Other..."}."SAM" ("Profile")) -> (x = y?=w290:bool)
          }
        }
        n201 = call "Display Message to User"("Enable"=w276) -> ("OK"=w275:bool)  [unwired: 9 in, 1 out]
        n202 = case shown="False" w275 {
          tunnel: [w287 w288] -> w272
          tunnel: "Vout  - Vbat profile" -> [w287 _]
          frame False {
          }
          frame True {
            w288 = enum16{"3.8VDC", "2.9VDC", "By Pass", "4.0VDC"}."2.9VDC" ("Vout  - Vbat profile")
            n203 = property on="Vout  - Vbat profile" class="Enum (strict)"("Value"=w288) -> ()  [unwired: 2 in, 2 out]
          }
        }
        n204 = case shown="\"4.0VDC\"" w272 {
          tunnel: [3.8 2.9 99.0 4.0] -> w268
          tunnel: [TRUE ("Visible") TRUE ("Visible") FALSE ("Visible") TRUE ("Visible")] -> _
          frame "3.8VDC", Default {
          }
          frame "2.9VDC" {
          }
          frame "By Pass" {
          }
          frame "4.0VDC" {
          }
        }
        n205 = Number To Fractional String(number=w268, width (-)=i16 1, precision (6)=i16 1) -> (F-format string=w271:string)  [unwired: 1 in]
        n206 = Concatenate Strings("LDO: " ("string"), w271, "V" ("string")) -> ()  [unwired: 1 out]
      }
      event "Internal PW": Value Change {
        n207 = event-data() -> ()  [unwired: 1 in, 6 out]
        n208 = local read "Sampling Rate"() -> (w295:T1)
        n209 = case shown="True" "Internal PW" {
          tunnel: [T6."Internal PW Source" ("Ex/Int PW") T6."External PW Source" ("Ex/Int PW")] -> w307
          frame False {
            # "Internal power source"
          }
          frame True {
            # "External Power Source"
          }
        }
        n210 = property on="Ext PW Vol Monitor" class="Bool (strict)"() -> ("Value"=w303:bool)  [unwired: 2 in, 2 out]
        n211 = property on="Range - Shunts" class="Enum (strict)"() -> ("Value"=w306:T2)  [unwired: 2 in, 2 out]
        n212 = local read "Task out"() -> (w310:refnum<k21>)
        n213 = local read "USB"() -> (w305:tag)
        n214 = call "Sample rate to sample collected.vi"("Sampling Rate _menu"=w295) -> ("Sample_rate"=w293:u32, "Sample"=w294:i32)  [unwired: 9 in]
        n215 = local write "Samples"(w294) -> ()
        n216 = call "UEvent_SET_INTERNAL_EXTERNAL_POWER_SOURCE.vi"("Ex/Int PW"=w307, "Sample rate"=w293, "Ext PW Vol Monitor"=w303, "USB"=w305, "Value"=w306, "Refnum in"=w310) -> ("External Voltage HIGH"=w302:bool, "Battery_Voltage"=w309:dbl, "DUT_Voltage"=w308:dbl, "Refnum out"=w304:refnum<k21>)  [unwired: 2 in]
        n217 = local read "Measure"() -> (w301:bool)
        n218 = case shown="True" w302 {
          tunnel: w302 -> [_ w318]
          tunnel: [w317 w318] -> w297
          tunnel: "Internal PW" -> [w317 _]
          frame True {
          }
          frame False {
            n219 = property on="Internal PW" class="Bool (strict)"("Value"=w318) -> ()  [unwired: 2 in, 2 out]
          }
        }
        n220 = local write "PW_Internal_Source"(w309) -> ()
        n221 = local write "Vbat"(w308) -> ()
        n222 = case shown="False" w301 {
          tunnel: w304 -> [_ w316]
          tunnel: [refnum<k21> "Stop" ("Refnum out") w316] -> w300
          frame False {
          }
          frame True {
          }
        }
        n223 = local read "Vout  - Vbat profile"() -> (w298:enum16{"3.8VDC", "2.9VDC", "By Pass", "4.0VDC"})
        n224 = local write "Task out"(w300) -> ()
        n225 = local write "EX_IN_INdicator"(w297) -> ()
        n226 = Not(x=w297) -> (.not. x?=w296:bool)
        n227 = case shown="\"By Pass\"" w298 {
          tunnel: w296 -> [w311 w312 _ w314]
          tunnel: [w311 w312 FALSE w314] -> _
          frame "3.8VDC", Default {
          }
          frame "2.9VDC" {
          }
          frame "By Pass" {
          }
          frame "4.0VDC" {
          }
        }
        "PW_Source" <- "Internal PW"
      }
      event "bypass Shunt": Value Change {
        n228 = event-data() -> ()  [unwired: 1 in, 6 out]
        n229 = Not(x="bypass Shunt") -> (.not. x?=w330:bool)
        n230 = local read "Sampling Rate"() -> (w322:T1)
        n231 = case shown="True" "bypass Shunt" {
          tunnel: [T7."Turn Off bypass - On Shunt" ("Bypass Shunt") T7."Turn On bypass - Off Shunt" ("Bypass Shunt")] -> w334
          frame False {
            # "add Shunt"
          }
          frame True {
            # "No Shunt"
          }
        }
        n232 = property on="schematic" class="Bool (strict)"("Value"=w330) -> ()  [unwired: 2 in, 2 out]
        n233 = property on="Ext PW Vol Monitor" class="Bool (strict)"() -> ("Value"=w328:bool)  [unwired: 2 in, 2 out]
        n234 = local read "Task out"() -> (w331:refnum<k21>)
        n235 = local read "USB"() -> (w333:tag)
        n236 = call "Sample rate to sample collected.vi"("Sampling Rate _menu"=w322) -> ("Sample_rate"=w321:u32, "Sample"=w323:i32)  [unwired: 9 in]
        n237 = local write "Samples"(w323) -> ()
        n238 = property on="Range - Shunts" class="Enum (strict)"() -> ("Value"=w332:T2)  [unwired: 2 in, 2 out]
        n239 = call "UEvent_SET_BYPASS_SHUNT_OR_NOT.vi"("Sample rate"=w321, "Task in"=w331, "Ext PW Vol Monitor"=w328, "USB"=w333, "Bypass Shunt"=w334, "Range_shunt"=w332) -> ("error out"=→"error out 3":errorcluster, "Task out"=w325:refnum<k21>)  [unwired: 4 in]
        n240 = local read "Measure"() -> (w327:bool)
        n241 = local write "Task out"(w325) -> ()
        n242 = case shown="False" w327 {
          tunnel: w325 -> [_ w336]
          tunnel: [refnum<k21> "Stop" ("Refnum out") w336] -> w326
          frame False {
          }
          frame True {
          }
        }
        n243 = local write "Task out"(w326) -> ()
      }
      event "Power ON/OFF": Value Change {
        n244 = event-data() -> ()  [unwired: 1 in, 6 out]
        n245 = case shown="False" "Power ON/OFF" {
          tunnel: [enum16{"Power ON DUT", "Power OFF DUT"}."Power OFF DUT" ("Power ON/OFF DUT") enum16{"Power ON DUT", "Power OFF DUT"}."Power ON DUT" ("Power ON/OFF DUT")] -> w351
          frame False {
          }
          frame True {
            # "ON"
          }
        }
        n246 = local read "Sampling Rate"() -> (w340:T1)
        n247 = local read "Vout  - Vbat profile"() -> (w350:enum16{"3.8VDC", "2.9VDC", "By Pass", "4.0VDC"})
        n248 = property on="Ext PW Vol Monitor" class="Bool (strict)"() -> ("Value"=w346:bool)  [unwired: 2 in, 2 out]
        n249 = property on="Range - Shunts" class="Enum (strict)"() -> ("Value"=w349:T2)  [unwired: 2 in, 2 out]
        n250 = local read "Task out"() -> (w353:refnum<k21>)
        n251 = local read "USB"() -> (w348:tag)
        n252 = call "Sample rate to sample collected.vi"("Sampling Rate _menu"=w340) -> ("Sample_rate"=w339:u32, "Sample"=w341:i32)  [unwired: 9 in]
        n253 = local write "Samples"(w341) -> ()
        n254 = call "UEvent_ON_OFF_POWER_SOURCE.vi"("Sample rate"=w339, "USB"=w348, "Power ON/OFF DUT"=w351, "Ext PW Vol Monitor"=w346, "Value"=w349, "Vout  - Vbat profile"=w350, "Refnum in"=w353) -> ("Battery_Voltage"=w352:dbl, "DUT_Voltage"=w342:dbl, "Refnum out"=w343:refnum<k21>)  [unwired: 2 in]
        n255 = local read "Measure"() -> (w345:bool)
        n256 = local write "PW_Internal_Source"(w352) -> ()
        n257 = local write "Vbat"(w342) -> ()
        n258 = local write "vbat_lb"(w342) -> ()
        n259 = local write "Task out"(w343) -> ()
        n260 = case shown="False" w345 {
          tunnel: w343 -> [_ w355]
          tunnel: [refnum<k21> "Stop" ("Refnum out") w355] -> w344
          frame False {
          }
          frame True {
          }
        }
        n261 = local write "Task out"(w344) -> ()
        "POWER ON_OFF" <- "Power ON/OFF"
      }
      event "Profile": Value Change {
        n262 = event-data() -> ()  [unwired: 1 in, 6 out]
        n263 = case shown="\"Hi-POWER\"" "Profile" {
          tunnel: [enum16{"3.8VDC", "2.9VDC", "By Pass", "4.0VDC"}."2.9VDC" ("DUT Voltage Selector") enum16{"3.8VDC", "2.9VDC", "By Pass", "4.0VDC"}."By Pass" ("DUT Voltage Selector") enum16{"3.8VDC", "2.9VDC", "By Pass", "4.0VDC"}."3.8VDC" ("DUT Voltage Selector") enum16{"3.8VDC", "2.9VDC", "By Pass", "4.0VDC"}."By Pass" ("DUT Voltage Selector")] -> w358
          frame "SAM", Default {
          }
          frame "Other..." {
          }
          frame "DIANA" {
          }
          frame "Hi-POWER" {
          }
        }
        n264 = local write "Vout  - Vbat profile"(w358) -> ()
      }
      event "Waveform_main": Cursor Move {
        n265 = event-data() -> ()  [unwired: 1 in, 9 out]
        n266 = local read "Waveform_main"() -> (w372:waveform(sgl))
        n267 = property on="Waveform_main" class="WFGraph (strict)"() -> ("CrsrList"=w382:T8)  [unwired: 2 in, 2 out]
        n268 = local read "Sampling Rate"() -> (w365:T1)
        n269 = call "Sample rate to sample collected.vi"("Sampling Rate _menu"=w365) -> ("Sample_rate"=w364:u32)  [unwired: 9 in, 1 out]
        n270 = call "uA_daq_Capture_Current_waveform_to_new_chart.vi"("Sample rate"=w364, "CrsrList"=w382, "Waveform_main"=w372) -> ("Numeric"=w379:dbl, "Waveform"=w380:waveform(sgl), "Numeric 2"=w381:sgl)  [unwired: 6 in]
        n271 = local write "Avg"(w381) -> ()
        n272 = local write "Waveform_sub"(w380) -> ()
        n273 = property on="Waveform_sub" class="WFGraph (strict)"("XScale.Maximum"=w379, "XScale.Minimum"=0.0 ("X Scale.Range:Minimum")) -> (error out=w366:errorcluster)  [unwired: 2 in, 1 out]
        n274 = property on="Waveform_main" class="WFGraph (strict)"(error in=w366, "Active Cursor"=u32 1) -> (error out=w374:errorcluster, "Value"=w373:waveform(sgl), "Cursor.Cursor X"=w376:dbl)  [unwired: 1 in, 1 out]
        n275 = property on="Waveform_main" class="WFGraph (strict)" props=["CrsrList", "Active Cursor", "Cursor", "Cursor X"](error in=w374, "Active Cursor"=u32 0) -> ("Cursor.Cursor X"=w375:dbl)  [unwired: 1 in, 3 out]
        n276 = call "uA_daq_calculate_All_values_from Sub_chart.vi"("Cursor.Cursor X 2"=w376, "Cursor.Cursor X"=w375, "Value"=w373, "Sample rate"=w364) -> ("Max value"=→"Max":dbl, "Average"=→"Avg":dbl, "Delta(s)"=→"Delta(s)":sgl, "Min value"=→"Min":dbl)  [unwired: 3 in, 1 out]
      }
      event "Calib": Value Change {
        w388 = Range_Shunt_selector."uA Range  Rs = 3.3ohm" ("Range - Shunts")
        n277 = event-data() -> ()  [unwired: 1 in, 6 out]
        n278 = call "Display Message to User2"() -> ("error out"=w384:errorcluster)  [unwired: 10 in, 1 out]
        n279 = flat-sequence {
          tunnel: w384 -> [_]
          tunnel: [w448] -> w386
          tunnel: [w443] -> w387
          frame #0 {
            n280 = local write "Measure"(FALSE ("Measure")) -> ()
          }
          frame #1 {
            n281 = local read "Task out"() -> (w443:refnum<k21>)
            n282 = local write "Waveform_main"(waveform(sgl) {"t0"=timestamp(0 s since 1904-01-01), "dt"=1.0, "Y"=[]} ("Waveform_main")) -> ()
            n283 = Wait (ms)(milliseconds to wait=u32 1000) -> ()  [unwired: 1 out]
            n284 = local write "uA_bank0"(0.0 ("uA_bank0")) -> ()
            n285 = call <vilib>:"DAQmx Stop Task.vi"("task/channels in"=w443) -> ("task out"=w445:refnum<k21>, "error out"=w446:errorcluster)  [unwired: 13 in]
            n286 = call <vilib>:"DAQmx Clear Task.vi"("task in"=w445, "error in"=w446) -> ("error out"=w444:errorcluster)  [unwired: 13 in]
            n287 = local read "USB"() -> (w448:tag)
            n288 = case shown="Error" w444 {
              frame No Error {
                n289 = local write "Task out"(refnum<k21> "Stop" ("y")) -> ()
              }
              frame Error {
              }
            }
          }
        }
        n290 = call "UEvent_MEASURE_FULL_PROCESS_START.vi"("Refnum in"=w387, "Range - Shunts"=w388, "Ext PW Vol Monitor"=FALSE, "USB"=w386, "Internal/external Power"=FALSE) -> ("Refnum out"=w390:refnum<k21>, "error out"=w391:errorcluster)  [unwired: 4 in, 5 out]
        n291 = while {
          tunnel: w391 -> [w435]
          tunnel: w390 -> [w437]
          tunnel: [w435] -> w389
          stop <- TRUE stop-if-true
          n292 = local write "Task out"(w437) -> ()
          n293 = local write "Measure"(TRUE ("Measure")) -> ()
          n294 = Wait (ms)(milliseconds to wait=u32 10000) -> ()  [unwired: 1 out]
        }
        n295 = flat-sequence {
          tunnel: w389 -> [w430]
          tunnel: w388 -> [w431]
          tunnel: [w430] -> w385
          frame #0 {
            n296 = local read "Average (uA)"() -> (w433:dbl)
            n297 = local read "DEV SN"() -> (w432:u32)
            n298 = local write "Measure"(FALSE ("Measure")) -> ()
            n299 = local write "uA_bank0"(w433) -> ()
            n300 = call "Calibration_Save_file.vi"("Current"=w433, "Range - Shunts"=w431, "DEV SN"=w432) -> ()  [unwired: 8 in, 1 out]
          }
        }
        n301 = flat-sequence {
          tunnel: w385 -> [w400]
          tunnel: [w400] -> w396
          tunnel: [w399] -> w395
          tunnel: [w398] -> w394
          tunnel: [Range_Shunt_selector."mA Range Rs = 1ohm" ("Range - Shunts")] -> w383
          tunnel: w396 -> [_]
          tunnel: w395 -> [w415]
          tunnel: w394 -> [w414]
          tunnel: w383 -> [w412]
          frame #0 {
            n302 = flat-sequence {
              tunnel: [w410] -> w398
              tunnel: [w405] -> w399
              frame #0 {
                n303 = local write "Measure"(FALSE ("Measure")) -> ()
                n304 = Wait (ms)(milliseconds to wait=u32 1000) -> ()  [unwired: 1 out]
              }
              frame #1 {
                n305 = local read "Task out"() -> (w405:refnum<k21>)
                n306 = local read "USB"() -> (w410:tag)
                n307 = local write "Waveform_main"(waveform(sgl) {"t0"=timestamp(0 s since 1904-01-01), "dt"=1.0, "Y"=[]} ("Waveform_main")) -> ()
                n308 = Wait (ms)(milliseconds to wait=u32 2000) -> ()  [unwired: 1 out]
                n309 = local write "mARange"(0.0 ("uA_bank0")) -> ()
                n310 = call <vilib>:"DAQmx Stop Task.vi"("task/channels in"=w405) -> ("task out"=w407:refnum<k21>, "error out"=w408:errorcluster)  [unwired: 13 in]
                n311 = call <vilib>:"DAQmx Clear Task.vi"("task in"=w407, "error in"=w408) -> ("error out"=w406:errorcluster)  [unwired: 13 in]
                n312 = case shown="No Error" w406 {
                  frame No Error {
                    n313 = local write "Task out"(refnum<k21> "Stop" ("y")) -> ()
                  }
                  frame Error {
                  }
                }
              }
            }
          }
          frame #1 {
            n314 = property on="Range - Shunts" class="Enum (strict)"("Value"=w412) -> ()  [unwired: 2 in, 2 out]
            n315 = call "UEvent_MEASURE_FULL_PROCESS_START.vi"("Refnum in"=w415, "Range - Shunts"=w412, "Ext PW Vol Monitor"=FALSE, "USB"=w414, "Internal/external Power"=TRUE) -> ("Refnum out"=w417:refnum<k21>, "error out"=w416:errorcluster)  [unwired: 4 in, 5 out]
            n316 = while {
              tunnel: w416 -> [w425]
              tunnel: w417 -> [w427]
              tunnel: [w425] -> w413
              stop <- TRUE stop-if-true
              n317 = local write "Task out"(w427) -> ()
              n318 = local write "Measure"(TRUE ("Measure")) -> ()
              n319 = Wait (ms)(milliseconds to wait=u32 5000) -> ()  [unwired: 1 out]
            }
            n320 = flat-sequence {
              tunnel: w413 -> [w420]
              tunnel: w412 -> [w421]
              frame #0 {
                n321 = local read "Average (uA)"() -> (w422:dbl)
                n322 = local write "Measure"(FALSE ("Measure")) -> ()
                n323 = local read "DEV SN"() -> (w423:u32)
                n324 = local write "mARange"(w422) -> ()
                n325 = call "Calibration_Save_file.vi"("Current"=w422, "error in (no error)"=w420, "Range - Shunts"=w421, "DEV SN"=w423) -> ()  [unwired: 7 in, 1 out]
              }
            }
          }
          frame #2 {
            n326 = call "Display Message to User3"() -> ()  [unwired: 10 in, 2 out]
          }
        }
      }
      event "Clear Graph": Value Change {
        n327 = event-data() -> ()  [unwired: 1 in, 6 out]
        n328 = flat-sequence {
          frame #0 {
            w450 = waveform(sgl) {"t0"=timestamp(0 s since 1904-01-01), "dt"=1.0, "Y"=[]} ("Waveform_main")
            n329 = local write "Clear"(TRUE ("Clear")) -> ()
            n330 = Wait (ms)(milliseconds to wait=u32 500) -> ()  [unwired: 1 out]
            n331 = local write "Waveform_main"(w450) -> ()
            n332 = local write "Waveform_sub"(w450) -> ()
          }
          frame #1 {
            n333 = local write "Clear"(FALSE ("Clear")) -> ()
          }
        }
      }
      event "ZOOM +": Value Change {
        n334 = event-data() -> ()  [unwired: 1 in, 6 out]
        n335 = property on="Waveform_main" class="WFGraph (strict)" props=["XScale", "Range", "XScale", "Increment", "XScale", "Maximum", "XScale", "Minimum"]() -> ("XScale.Maximum"=w459:dbl, "XScale.Minimum"=w455:dbl)  [unwired: 2 in, 4 out]
        n336 = Subtract(x=w459, y=0.1) -> (x-y=w457:dbl)
        n337 = Add(x=w455, y=0.1) -> (x+y=w454:dbl)
        n338 = property on="Waveform_main" class="WFGraph (strict)"("XScale.Maximum"=w457, "XScale.Minimum"=w454) -> ()  [unwired: 2 in, 2 out]
      }
      event "ZOOM -": Value Change {
        n339 = event-data() -> ()  [unwired: 1 in, 6 out]
        n340 = property on="Waveform_main" class="WFGraph (strict)" props=["XScale", "Range", "XScale", "Increment", "XScale", "Maximum", "XScale", "Minimum"]() -> ("XScale.Maximum"=w468:dbl, "XScale.Minimum"=w464:dbl)  [unwired: 2 in, 4 out]
        n341 = Add(x=w468, y=0.1) -> (x+y=w466:dbl)
        n342 = Subtract(x=w464, y=0.1) -> (x-y=w461:dbl)
        n343 = Less Than 0?(x=w461) -> (x < 0?=w463:bool)
        n344 = Select(t=0.0, s=w463, f=w461) -> (s? t:f=w460:dbl)
        n345 = property on="Waveform_main" class="WFGraph (strict)"("XScale.Maximum"=w466, "XScale.Minimum"=w460) -> ()  [unwired: 2 in, 2 out]
      }
      event "ZOOM M1M2": Value Change {
        n346 = event-data() -> ()  [unwired: 1 in, 6 out]
        n347 = property on="Waveform_main" class="WFGraph (strict)"("Active Cursor"=u32 0) -> (error out=w475:errorcluster)  [unwired: 2 in, 1 out]
        n348 = property on="Waveform_main" class="WFGraph (strict)"(error in=w475) -> (error out=w472:errorcluster, "Cursor.Cursor X"=w470:dbl)  [unwired: 1 in, 1 out]
        n349 = property on="Waveform_main" class="WFGraph (strict)"(error in=w472, "Active Cursor"=u32 1) -> (error out=w474:errorcluster)  [unwired: 1 in, 1 out]
        n350 = property on="Waveform_main" class="WFGraph (strict)"(error in=w474) -> ("Cursor.Cursor X"=w469:dbl)  [unwired: 1 in, 2 out]
        n351 = Greater?(x=w470, y=w469) -> (0:w471:bool)
        n352 = case shown="True" w471 {
          tunnel: w470 -> [w478 w480]
          tunnel: w469 -> [w477 w479]
          frame False {
            n353 = property on="Waveform_main" class="WFGraph (strict)"("XScale.Maximum"=w477, "XScale.Minimum"=w478) -> ()  [unwired: 2 in, 2 out]
          }
          frame True {
            n354 = property on="Waveform_main" class="WFGraph (strict)"("XScale.Maximum"=w480, "XScale.Minimum"=w479) -> ()  [unwired: 2 in, 2 out]
          }
        }
      }
      event "Center": Value Change {
        n355 = event-data() -> ()  [unwired: 1 in, 6 out]
        n356 = property on="Waveform_main" class="WFGraph (strict)"() -> ("XScale.Maximum"=w485:dbl, "XScale.Minimum"=w484:dbl)  [unwired: 2 in, 2 out]
        n357 = Add(x=w485, y=w484) -> (x+y=w483:dbl)
        n358 = Divide(x=w483, y=2.0) -> (x/y=w481:dbl)
        n359 = property on="Waveform_main" class="WFGraph (strict)" props=["Value", "Active Cursor", "Cursor", "Cursor X"]("Active Cursor"=u32 1, "Cursor.Cursor X"=w481) -> (error out=w486:errorcluster)  [unwired: 2 in, 2 out]
        n360 = property on="Waveform_main" class="WFGraph (strict)" props=["CrsrList", "Active Cursor", "Cursor", "Cursor X"](error in=w486, "Active Cursor"=u32 0, "Cursor.Cursor X"=w481) -> ()  [unwired: 1 in, 3 out]
      }
      event "stop": Value Change {
        n361 = event-data() -> ()  [unwired: 1 in, 6 out]
        n362 = flat-sequence {
          tunnel: [w493] -> w489
          tunnel: w489 -> [w502]
          frame #0 {
            n363 = local write "Task out"(refnum<k21> "Stop" ("Task out")) -> ()
          }
          frame #1 {
            n364 = local read "USB"() -> (w501:tag)
            n365 = local read "Task out"() -> (w496:refnum<k21>)
            n366 = call "uA_daq_Set_Relay_internal_power_on_off_from_baterry.vi"("Power ON/OFF DUT"=enum16{"Power ON DUT", "Power OFF DUT"}."Power OFF DUT", "USB DAQ"=w501) -> ("error out"=w492:errorcluster)  [unwired: 9 in]
            n367 = call <vilib>:"DAQmx Stop Task.vi"("task/channels in"=w496, "error in"=w492) -> ("task out"=w491:refnum<k21>, "error out"=w494:errorcluster)  [unwired: 12 in]
            n368 = call <vilib>:"DAQmx Clear Task.vi"("task in"=w491, "error in"=w494) -> ("error out"=w495:errorcluster)  [unwired: 13 in]
            n369 = local read "USB"() -> (w499:tag)
            n370 = call <vilib>:"Clear Errors.vi"("error in (no error)"=w495) -> ("error out"=w498:errorcluster)  [unwired: 5 in, 1 out]
            n371 = call "uA_daq_ON_OFF_LED_Measure.vi"("error in"=w498, "LED_meas"=FALSE ("Boolean"), "USB"=w499) -> ("error out"=w493:errorcluster)  [unwired: 8 in]
          }
          frame #2 {
            n372 = local read "Ver"() -> (w503:string)
            n373 = call <vilib>:"Clear Errors.vi"("error in (no error)"=w502) -> ()  [unwired: 5 in, 2 out]
            n374 = Empty String/Path?(string/path=w503) -> (empty?=w504:bool)
            n375 = case shown="False" w504 {
              frame True {
              }
              frame False {
                n376 = Quit LabVIEW(quit? (T)=TRUE) -> ()
              }
            }
          }
          frame #3 {
            n377 = Stop(stop? (T)=TRUE) -> ()
          }
        }
      }
      event "Save": Value Change {
        n378 = event-data() -> ()  [unwired: 1 in, 6 out]
        n379 = local read "Waveform_main"() -> (w508:waveform(sgl))
        n380 = call "File Dialog"("pattern (all files)"="*.dlog", "pattern label"="datalog") -> ("selected path"=w511:path)  [unwired: 10 in, 3 out]
        n381 = call-poly <vilib>:"Write Waveforms to File.vi"("append to file? (new file:F)"=FALSE, "waveform"=w508, "file path (dialog if empty)"=w511) -> ()  [unwired: 7 in, 2 out]
      }
      event "Load": Value Change {
        (unwired) FALSE ("append to file? (new file:F)")
        n382 = event-data() -> ()  [unwired: 1 in, 6 out]
        n383 = call "File Dialog3"("pattern (all files)"="*.dlog", "pattern label"="datalog") -> ("selected path"=w515:path)  [unwired: 10 in, 3 out]
        n384 = call-poly <vilib>:"Read Waveforms from File.vi"("file path (dialog if empty)"=w515) -> ("first waveform in record"=w512:waveform(dbl))  [unwired: 5 in, 3 out]
        n385 = local write "Waveform_main"(w512) -> ()
      }
      event "Take Picture": Value Change {
        n386 = event-data() -> ()  [unwired: 1 in, 6 out]
        n387 = call <vilib>:"Application Directory.vi"() -> ("Application Directory"=w517:path)
        n388 = control-ref of="This VI"() -> (w521:refnum<vi>)
        n389 = call "File Dialog2"("start path"=w517, "pattern (all files)"="*.jpg", "pattern label"="*.jpg") -> ("selected path"=w523:path, "error out"=w520:errorcluster)  [unwired: 9 in, 2 out]
        n390 = invoke on="Invoke Node" class="VI" method="FP.Get Image"(reference=w521, "image depth"=enum32{"File", "Clipboard"}."File" ("Target")) -> ("image data"=w522:T9)  [unwired: 4 in, 5 out]
        n391 = call <vilib>:"Clear Errors.vi"("error in (no error)"=w520) -> ()  [unwired: 5 in, 2 out]
        n392 = call <vilib>:"Write JPEG File.vi"("image data"=w522, "path to JPEG file"=w523) -> ()  [unwired: 8 in, 2 out]
      }
      event "Save setting": Value Change {
        w545 = "SETTING" ("section")
        n393 = event-data() -> ()  [unwired: 1 in, 6 out]
        n394 = call <vilib>:"Application Directory.vi"() -> ("Application Directory"=w550:path)
        n395 = local read "Range - Shunts"() -> (w538:T2)
        n396 = Build Path(base path=w550, name or relative path="Setting.cfg") -> (appended path=w548:path)
        n397 = local read "Vout  - Vbat profile"() -> (w535:enum16{"3.8VDC", "2.9VDC", "By Pass", "4.0VDC"})
        n398 = call <vilib>:"Open Config Data.vi"("create file if necessary (T)"=TRUE, "configuration file path"=w548) -> ("error out"=w524:errorcluster, "refnum"=w546:T5)  [unwired: 7 in, 1 out]
        n399 = local read "Profile"() -> (w537:enum16{"SAM", "DIANA", "Hi-POWER", "Other..."})
        n400 = call-poly <vilib>:"Write Key.vi"("section"=w545, "error in (no error)"=w524, "value"=w538, "key"="Range - Shunts", "refnum"=w546) -> ("error out"=w525:errorcluster, "refnum out"=w543:T5)  [unwired: 4 in, 1 out]
        n401 = local read "Internal PW"() -> (w533:bool)
        n402 = call-poly <vilib>:"Write Key.vi"("section"=w545, "error in (no error)"=w525, "value"=w537, "key"="Profile", "refnum"=w543) -> ("error out"=w526:errorcluster, "refnum out"=w544:T5)  [unwired: 4 in, 1 out]
        n403 = local read "bypass Shunt"() -> (w531:bool)
        n404 = call-poly <vilib>:"Write Key.vi"("section"=w545, "error in (no error)"=w526, "value"=w535, "key"="Vout  - Vbat profile", "refnum"=w544) -> ("error out"=w527:errorcluster, "refnum out"=w542:T5)  [unwired: 4 in, 1 out]
        n405 = call-poly <vilib>:"Write Key.vi"("section"=w545, "error in (no error)"=w527, "value"=w533, "key"="Internal PW", "refnum"=w542) -> ("error out"=w528:errorcluster, "refnum out"=w541:T5)  [unwired: 4 in, 1 out]
        n406 = call-poly <vilib>:"Write Key.vi"("section"=w545, "error in (no error)"=w528, "value"=w531, "key"="bypass Shunt", "refnum"=w541) -> ("error out"=w529:errorcluster, "refnum out"=w530:T5)  [unwired: 4 in, 1 out]
        n407 = call <vilib>:"Close Config Data.vi"("error in (no error)"=w529, "refnum"=w530) -> ()  [unwired: 8 in, 2 out]
      }
    }
  }
  n408 = while {
    tunnel: w4 -> [w560]
    tunnel: [w559] -> w7
    shift-right: [w555] -> w6
    shift-left: w5 -> [w557]
    stop <- FALSE ("stop (F)") stop-if-true
    n409 = local read "Range - Shunts"() -> (w554:T2)
    n410 = local read "Samples"() -> (w551:i32)
    n411 = Equal?(x=w557, y=refnum<k21> "Stop") -> (x = y?=w553:bool)
    n412 = case shown="False" w553 {
      tunnel: w560 -> [w563 w571]
      tunnel: [w563 w570] -> w559
      tunnel: w557 -> [_ w567]
      tunnel: [w562 w569] -> w555
      tunnel: w554 -> [_ w568]
      tunnel: refnum<k21> refnum ("task out") -> [_ w565]
      tunnel: w551 -> [_ w564]
      frame True {
        n413 = Wait (ms)(milliseconds to wait=u32 100) -> ()  [unwired: 1 out]
        n414 = local read "Task out"() -> (w562:refnum<k21>)
      }
      frame False {
        n415 = Not Equal?(x=w567, y=w565) -> (x != y?=w566:bool)
        n416 = case shown="True" w566 {
          tunnel: w571 -> [w573 w579]
          tunnel: [w573 w578] -> w570
          tunnel: w567 -> [_ w577]
          tunnel: [w572 w576] -> w569
          tunnel: w568 -> [_ w575]
          tunnel: w564 -> [_ w574]
          frame False {
            n417 = local read "Task out"() -> (w572:refnum<k21>)
          }
          frame True {
            n418 = case shown="\"mA Range Rs = 1ohm\"" w575 {
              tunnel: w579 -> [w586 w597 w608 w619]
              tunnel: [w585 w596 w607 w618] -> w578
              tunnel: w577 -> [w584 w595 w606 w617]
              tunnel: [w583 w594 w605 w616] -> w576
              tunnel: w574 -> [w580 w591 w602 w613]
              frame "mA Range Rs = 1ohm" {
                n419 = call "DAQ_ADC_Max_Sample_Rate_For_USB_6001.vi"("number of samples per channel"=w580, "Refnum in"=w584) -> ("error out"=w582:errorcluster, "data"=w581:waveform(dbl))  [unwired: 8 in]
                n420 = case shown="No Error" w582 {
                  selector: w582 -> [_ w590]
                  tunnel: w586 -> [w589 _]
                  tunnel: [w588 _] -> w585
                  tunnel: w581 -> [w587 _]
                  frame No Error {
                    n421 = Enqueue Element(queue=w589, element=w587) -> (queue out=w588:refnum<queue>)  [unwired: 2 in, 2 out]
                  }
                  frame Error {
                    n422 = call <vilib>:"Clear Errors.vi"("error in (no error)"=w590) -> ()  [unwired: 5 in, 2 out]
                  }
                }
                n423 = local read "Task out"() -> (w583:refnum<k21>)
              }
              frame "mA Range Rs = 1ohm - X2" {
                n424 = call "DAQ_ADC_Max_Sample_Rate_For_USB_6001.vi"("number of samples per channel"=w591, "Refnum in"=w595) -> ("error out"=w593:errorcluster, "data"=w592:waveform(dbl))  [unwired: 8 in]
                n425 = case shown="No Error" w593 {
                  selector: w593 -> [_ w601]
                  tunnel: w597 -> [w600 _]
                  tunnel: [w599 _] -> w596
                  tunnel: w592 -> [w598 _]
                  frame No Error {
                    n426 = Enqueue Element(queue=w600, element=w598) -> (queue out=w599:refnum<queue>)  [unwired: 2 in, 2 out]
                  }
                  frame Error {
                    n427 = call <vilib>:"Clear Errors.vi"("error in (no error)"=w601) -> ()  [unwired: 5 in, 2 out]
                  }
                }
                n428 = local read "Task out"() -> (w594:refnum<k21>)
              }
              frame "mA Range Rs = 3.3ohm" {
                n429 = call "DAQ_ADC_Max_Sample_Rate_For_USB_6001.vi"("number of samples per channel"=w602, "Refnum in"=w606) -> ("error out"=w604:errorcluster, "data"=w603:waveform(dbl))  [unwired: 8 in]
                n430 = case shown="No Error" w604 {
                  selector: w604 -> [_ w612]
                  tunnel: w608 -> [w611 _]
                  tunnel: [w610 _] -> w607
                  tunnel: w603 -> [w609 _]
                  frame No Error {
                    n431 = Enqueue Element(queue=w611, element=w609) -> (queue out=w610:refnum<queue>)  [unwired: 2 in, 2 out]
                  }
                  frame Error {
                    n432 = call <vilib>:"Clear Errors.vi"("error in (no error)"=w612) -> ()  [unwired: 5 in, 2 out]
                  }
                }
                n433 = local read "Task out"() -> (w605:refnum<k21>)
              }
              frame "uA Range  Rs = 3.3ohm" {
                n434 = call "DAQ_ADC_Max_Sample_Rate_For_USB_6001.vi"("number of samples per channel"=w613, "Refnum in"=w617) -> ("error out"=w615:errorcluster, "data"=w614:waveform(dbl))  [unwired: 8 in]
                n435 = case shown="No Error" w615 {
                  selector: w615 -> [_ w623]
                  tunnel: w619 -> [w622 _]
                  tunnel: [w621 _] -> w618
                  tunnel: w614 -> [w620 _]
                  frame No Error {
                    n436 = Enqueue Element(queue=w622, element=w620) -> (queue out=w621:refnum<queue>)  [unwired: 2 in, 2 out]
                  }
                  frame Error {
                    n437 = call <vilib>:"Clear Errors.vi"("error in (no error)"=w623) -> ()  [unwired: 5 in, 2 out]
                  }
                }
                n438 = local read "Task out"() -> (w616:refnum<k21>)
              }
            }
          }
        }
      }
    }
  }
  n439 = while {
    tunnel: w4 -> [w629]
    tunnel: w1 -> [_]
    stop <- FALSE stop-if-true
    n440 = property on="Ext PW Vol Monitor" class="Bool (strict)"() -> ("Value"=w635:bool)  [unwired: 2 in, 2 out]
    n441 = property on="Range - Shunts" class="Enum (strict)"() -> ("Value"=w633:T2)  [unwired: 2 in, 2 out]
    n442 = Get Queue Status(queue=w629) -> (queue out=w626:refnum<queue>, error out=w630:errorcluster, # elements in queue=w628:i32)  [unwired: 2 in, 5 out]
    n443 = Dequeue Element(queue=w629, error in (no error)=w630) -> (element=w634:waveform(sgl))  [unwired: 1 in, 3 out]
    n444 = local read "Waveform_main"() -> (w637:waveform(sgl))
    n445 = Greater?(x=w628, y=100) -> (0:w625:bool)
    n446 = case shown="\"mA Range Rs = 1ohm\"" w633 {
      tunnel: w634 -> [w649 w653 w657 w661]
      tunnel: [w646 w650 w654 w658] -> w632
      frame "mA Range Rs = 3.3ohm" {
        (unwired) 0.0 ("uA_bank0")
        n447 = call-poly <vilib>:"Basic Averaged DC-RMS.vi"("signal in"=w649) -> ("RMS value"=w647:dbl)  [unwired: 7 in, 3 out]
        n448 = Greater?(x=w647, y=3.5) -> (0:w646:bool)
      }
      frame "uA Range  Rs = 3.3ohm" {
        n449 = call-poly <vilib>:"Basic Averaged DC-RMS.vi"("signal in"=w653) -> ("RMS value"=w651:dbl)  [unwired: 7 in, 3 out]
        n450 = Greater?(x=w651, y=3.5) -> (0:w650:bool)
      }
      frame "mA Range Rs = 1ohm" {
        (unwired) 0.0 ("uA_bank0")
        n451 = call-poly <vilib>:"Basic Averaged DC-RMS.vi"("signal in"=w657) -> ("RMS value"=w655:dbl)  [unwired: 7 in, 3 out]
        n452 = Greater?(x=w655, y=4.0) -> (0:w654:bool)
      }
      frame "mA Range Rs = 1ohm - X2" {
        (unwired) 0.0 ("uA_bank0")
        n453 = call-poly <vilib>:"Basic Averaged DC-RMS.vi"("signal in"=w661) -> ("RMS value"=w659:dbl)  [unwired: 7 in, 3 out]
        n454 = Greater?(x=w659, y=2.0) -> (0:w658:bool)
      }
    }
    n455 = case shown="True" w625 {
      tunnel: w626 -> [_ w645]
      frame False {
      }
      frame True {
        n456 = Flush Queue(queue=w645) -> ()  [unwired: 1 in, 3 out]
      }
    }
    n457 = case shown="False" w635 {
      tunnel: w634 -> [w669 w678]
      tunnel: [w669 w677] -> w624
      tunnel: w632 -> [_ w675]
      tunnel: [FALSE w675] -> w631
      frame True {
        n458 = Unbundle By Name(w669) -> ("Y"=w668:sgl[])
        n459 = Add Array Elements(numeric array=w669) -> (sum=w666:sgl)
        n460 = Array Size(array=w668) -> (size(s)=w667:i32)
        n461 = Divide(x=w666, y=w667) -> (x/y=w663:sgl)
        n462 = Greater?(x=w663, y=6) -> (0:w665:bool)
        n463 = case shown="True" w665 {
          frame False {
          }
          frame True {
            n464 = property on="Internal PW" class="Bool (strict)"("Value"=TRUE ("Internal PW")) -> ()  [unwired: 2 in, 2 out]
            n465 = local read "USB"() -> (w672:tag)
            n466 = call "uA_daq_switch_external_internal_pw_source.vi"("USB DAQ"=w672, "Ex/Int PW"=T6."External PW Source") -> ()  [unwired: 9 in, 1 out]
          }
        }
      }
      frame False {
        n467 = property on="Range - Shunts" class="Enum (strict)"() -> ("Value"=w676:T2)  [unwired: 2 in, 2 out]
        n468 = local read "uA_bank0"() -> (w674:dbl)
        n469 = local read "mARange"() -> (w673:dbl)
        n470 = call "uA_daq_gain_caculator.vi"("Waveform Chart in"=w678, "Calib_value_ uA"=w674, "Calib_mA"=w673, "Range - Shunts"=w676) -> ("Waveform out"=w677:waveform(dbl))  [unwired: 11 in]
      }
    }
    n471 = local read "Measure"() -> (w636:bool)
    n472 = property on="out_range" class="Bool (strict)"("Visible"=w631) -> ()  [unwired: 2 in, 2 out]
    n473 = case shown="True" w636 {
      tunnel: w624 -> [_ w643]
      tunnel: w637 -> [_ w644]
      frame False {
      }
      frame True {
        n474 = call "WDT Append Waveforms SGL.vi"("waveform B"=w644, "waveform A"=w643) -> ("waveform out"=→"Waveform_main":waveform(sgl))  [unwired: 8 in, 1 out]
        n475 = local read "Waveform_main"() -> (w641:waveform(sgl))
        n476 = property on="Waveform_main" class="WFGraph (strict)"() -> ("CrsrList"=w642:T8)  [unwired: 2 in, 2 out]
        n477 = call "uA_daq_capture_small_curr_waveform.vi"("CrsrList"=w642, "Waveform_main"=w641) -> ("Numeric"=→"Average (uA)":sgl)  [unwired: 9 in]
      }
    }
  }
  n478 = Release Queue(queue=w7) -> ()  [unwired: 2 in, 3 out]
  n479 = call <vilib>:"DAQmx Clear Task.vi"("task in"=w6) -> ()  [unwired: 14 in, 1 out]
